vi "Host.vi"() -> ()   [LabVIEW 2018]
uses:
  <instrlib>/niDCPower/nidcpower.llb/niDCPower Measurement Type.ctl
  <vilib>/FPGAPlugInAG/PXI-7953R/niLvFpga_Open_PXI-7953R.vi
  <vilib>/rvi/interface/common/dynamic/niFpgaDynamicAddResources.vi
  <vilib>/FPGAPlugInAG/Dynamic/niLvFpga_Reset_Dynamic.vi
  <vilib>/FPGAPlugInAG/Dynamic/niLvFpga_Run_Dynamic.vi
  <vilib>/Utility/error.llb/Error Cluster From Error Code.vi
  <vilib>/rvi/errors/niLvFpgaAdjustHostInterfaceError.vi
  <vilib>/FPGAPlugInAG/Dynamic/niLvFpga_Close_Dynamic.vi
  <vilib>/rvi/interface/nirviOpenFPGA/nirviOpenFPGA.xnode
  FPGA Bitfiles/EV76C661aab_FPGATarget_Target_Ci7Vxfb6PyU.lvbitx
  <vilib>/rvi/interface/nirviMethod/nirviMethod.xnode
  <vilib>/rvi/interface/nirviReadWriteControl/nirviReadWriteControl.xnode
  <vilib>/rvi/interface/nirviCloseFPGA/nirviCloseFPGA.xnode
  NiFpgaLv.dll
  <vilib>/rvi/interface/Simulation/niFpgaSimulationCallBeginRW.vi
  <vilib>/FPGAPlugInAG/Dynamic/niLvFpga_ReadFifo_Dynamic.vi
  <vilib>/rvi/errors/niLvFpgaMergeErrorWithErrorCode.vi
panel:
  in  "Tab Control":enum32{"Панель управления", "Панель отладки"}(tab)
  in  "Frames":path=path "D:/NI LabVIEW/EV76C661_aab/Frames"
  out "CountFIFO":u32
  out "AddCounter":u32
  in  "Сохранить":bool
  in  "Темный(F)\nСветлый(T)":bool
  in  "Примечание":string
  out "Image":T1(plugin-control)
  in  "Непрерывно":bool
  in  "Получить кадр":bool
  out "Last SEU Time":string
  out "Reg Counter":u8
  in  "SEU":path=path "D:/NI LabVIEW/EV76C661_aab/SEU"
  out "Счетчик сбоев":u16
  in  "Содержание всех регистров":u16[](array[numeric])=[1, 0, 0, 0, 32880, 0, 53338, 2561, 56097, 24869, 512, 260, 0, 0, 512, 0, 0, 0, 6, 1024, 6, 1280, 0, 0, 0, 0, 0, 512, 0, 0, 0, 6, 1024, 6, 1280, 0, 512, 0, 0, 0, 6, 1024, 6, 1280, 0, 512, 0, 0, 0, 6, 1024, 6, 1280, 0, 32896, 32896, 0, 14464, 32960, 0, 0, 0, 0, 0, 0, 0, 0, 0, 8192, 0, 0, 0, 0, 31601, 0, 0, 0, 0, 0, 0, 0, 0, 0, 0, 0, 0, 0, 0, 0, 0, 0, 0, 0, 0, 0, 0, 0, 0, 0, 0, 0, 0, 0, 0, 0, 0, 0, 0, 0, 0, 0, 0, 0, 0, 0, 0, 0, 0, 0, 0, 0, 0, 0, 0, 0, 0, 0, 2048]
  in  "Регистры для записи":u16[](array[numeric])=[2561, 56217, 24976, 512, 260, 512]
  in  "Проверка\nсбоев":bool
  in  "Прошить\nрегистры":bool
  in  "TRIG":bool
  in  "Автомат":bool
  in  "SIM_SEL":bool
  in  "VDD18D_selcur, A":dbl=0.06 caption="current limit" format="%_6p"
  in  "VDD18A_selcur, A":dbl=0.05 caption="current limit" format="%_6p"
  in  "VDD33A_selcur, A":dbl=0.06 caption="current limit" format="%_6p"
  out "VDD18A_counter":u32
  out "VDD33A_counter":u32
  out "VDD18D_counter":u32
  out "VDD18A_SEL_warning":bool
  out "VDD33A_SEL_warning":bool
  out "VDD18D_SEL_warning":bool
  in  "STOP":bool
  in  "Power":bool
  in  "VDD18D, V":dbl=1.8 caption="voltage level" format="%_6p"
  in  "VDD18D_curlim, A":dbl=0.1 caption="current limit" format="%_6p"
  in  "VDD18A_curlim, A":dbl=0.1 caption="current limit" format="%_6p"
  out "VDD18D_cur, A":dbl caption="measurement" format="%_6g"
  out "VDD18A_cur, A":dbl caption="measurement" format="%_6g"
  in  "VDD18A, V":dbl=1.7999999999999985 caption="voltage level" format="%_6p"
  out "VDD18D_char":dbl(graph)=-0.006831291044701817
  out "VD18A_char":dbl(graph)=-2.772283562549262e-06
  in  "VDD33A_curlim, A":dbl=0.1 caption="current limit" format="%_6p"
  out "VDD33A_cur, A":dbl caption="measurement" format="%_6g"
  in  "VDD33A, V":dbl=3.300000000000001 caption="voltage level" format="%_6p"
  out "VDD18A_char":dbl(graph)=4.6397717644130316e-05
  in  "VDD33A_VDD18A":refnum<k15>="PXI1Slot2_2"
  in  "VDD18D":refnum<k15>="PXI1Slot3_3"
  in  "FPGA":tag="RIO0"
  in  "SEL":path=path "D:/NI LabVIEW/EV76C661_aab/SEL"
  out "№":string
  out "Default":string
  out "During SEU":string
  in  "Кадр готов":bool
  out "MISO":bool[](array[boolean])
  out "DataTime":u32
  out "DelayFrame":u32
  in  "WatchDogTime":u32=5000
  out "DataFailure":bool
  out "MOSI":bool[](array[boolean])
  out "Образец №":string="1"
  in  "NumberOfAdd":u32=1310720
  out "DataToFrame":u16[][](array[numeric])
  out "SEL":bool
  out "Сбой":bool
  in  "CSN в конце по С(F)/Ф(T)":bool
  in  "Чтение по С(F)/Ф(T)":bool=TRUE
  in  "Маска номера":i32[](array[numeric])=[0, -1, 2, 3, 4, 5, 6, 7, 8, 9, 10, 11, 12, 13, 14, 15, 16, 17, 18, 19, 20, 21, 22, 23, 24, 25, 26, 27, 28, 29, 30, 31, 32, 33, 34, 35, 36, 37, 38, 39, 40, 41, 42, 43, 44, 45, 46, 47, 48, 49, 50, 51, 52, 53, 54, 55, 56, 57, 58, 59, -1, -1, -1, -1, -1, -1, -1, -1, -1, -1, -1, -1, -1, -1, -1, -1, -1, -1, -1, -1, -1, -1, -1, -1, -1, -1, -1, -1, -1, -1, -1, -1, -1, -1, -1, -1, -1, -1, -1, -1, -1, -1, -1, -1, -1, -1, -1, -1, -1, -1, -1, -1, -1, -1, -1, -1, -1, -1, -1, -1, -1, -1, -1, -1, -1, -1, -1, 127, 0, 0, 0, 0, 0, 0, 0, 0, 0, 0, 0, 0, 0, 0, 0, 0, 0, 0, 0, 0, 0, 0, 0, 0, 0, 0, 0, 0, 0, 0, 0, 0, 0, 0, 0, 0, 0, 0, 0, 0, 0, 0, 0, 0, 0, 0, 0, 0, 0, 0, 0, 0, 0, 0, 0, 0, 0, 0, 0, 0, 0, 0, 0, 0, 0, 0, 0, 0, 0, 0, 0, 0, 0, 0, 0, 0, 0, 0, 0, 0, 0, 0, 0, 0, 0, 0, 0, 0, 0, 0, 0, 0, 0, 0, 0, 0, 0, 0, 0, 0, 0, 0, 0, 0, 0, 0, 0, 0, 0, 0, 0, 0, 0, 0, 0, 0, 0, 0, 0, 0, 0, 0, 0, 0, 0, 0, 0, 0]
  in  "Номера для Записи":u32[](array[numeric])=[7, 8, 9, 10, 11, 14]
  in  "Такт чтения после адреса":u8=1
  in  "27_STOP":u8=27
  in  "19_STOP":u8=19
  out "Power OFF":bool
  in  "Делитель 24/x":u8=2
  in  "RESET":bool
  in  "Wait_parry, ms":u32=100
  in  "VDD33_ON":bool
  in  "VDD18_ON":bool
  in  "TrigTime":u32=500
  in  "Retrieve":u8
  in  "Request":u8
  out "SPI":bool
  in  "SPI_Write":bool
  out "WriteIsDone":bool
  in  "SPI_Read":bool
  out "DataRead":u16
  in  "RegForRead":u8
  in  "RegForWrite":u8
  in  "DataWrite":u16
  out "ReadIsDone":bool
  out "FirmwareIsDone":bool
  # "0 - 7       h07\n1 - 8       h08\n2 - 9       h09\n3 - 10     h0A\n4 - 11     h0B\n5 - 14     h0E"
  # "h08\n56217\n56319"
  # "h09\n24960\n24976"
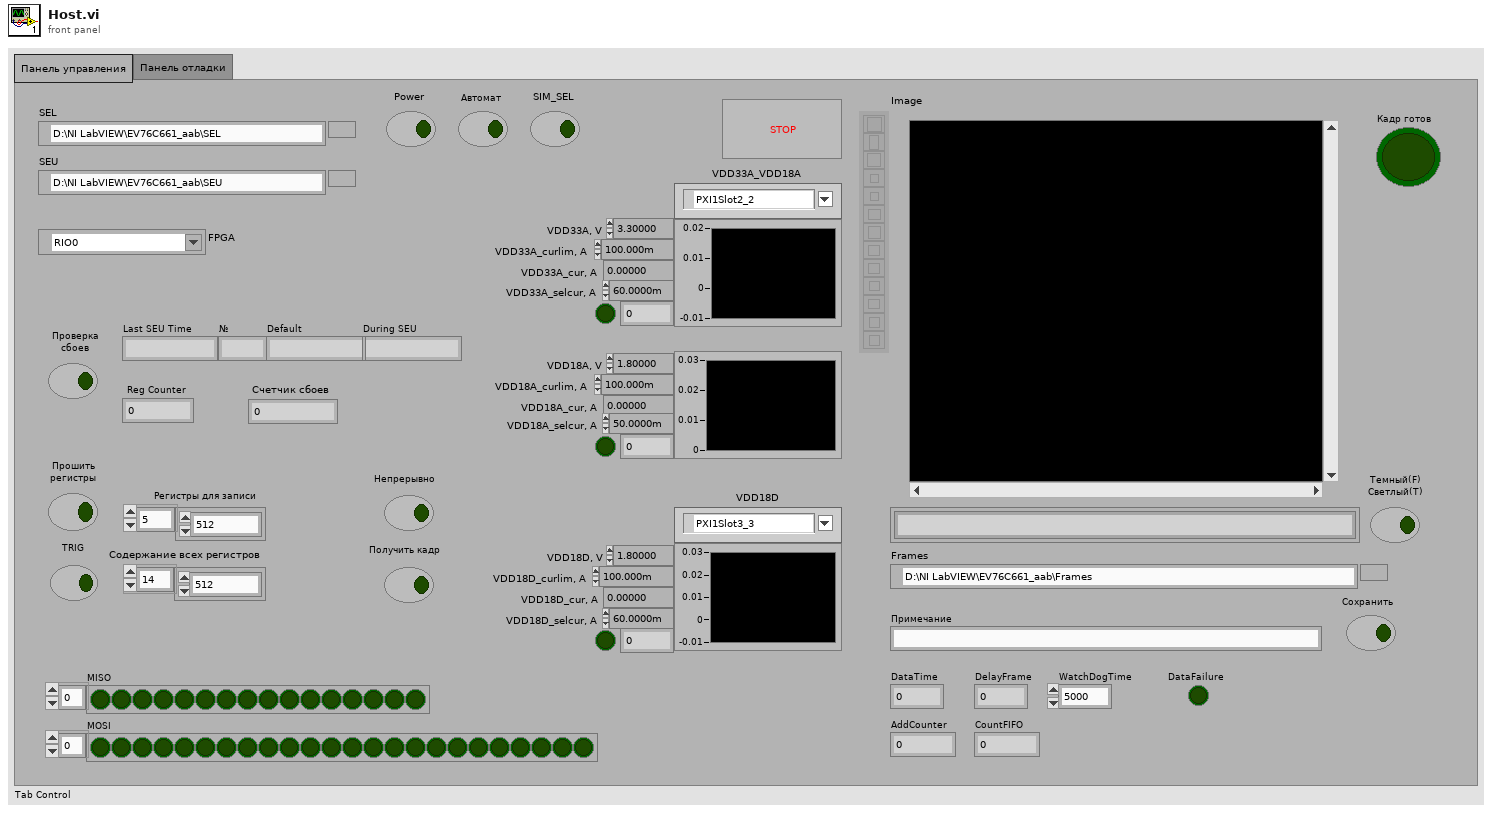
[diagram p1: front panel]
types:
  T1 = typedef "IMAQ Image.ctl" = refnum<image>
  T2 = enum16{"open", "replace", "create", "open or create", "replace or create", "replace or create with confirmation"}
  T3 = typedef "Image Type" = u32
  T4 = typedef "niDCPower Measurement Type.ctl" = i32
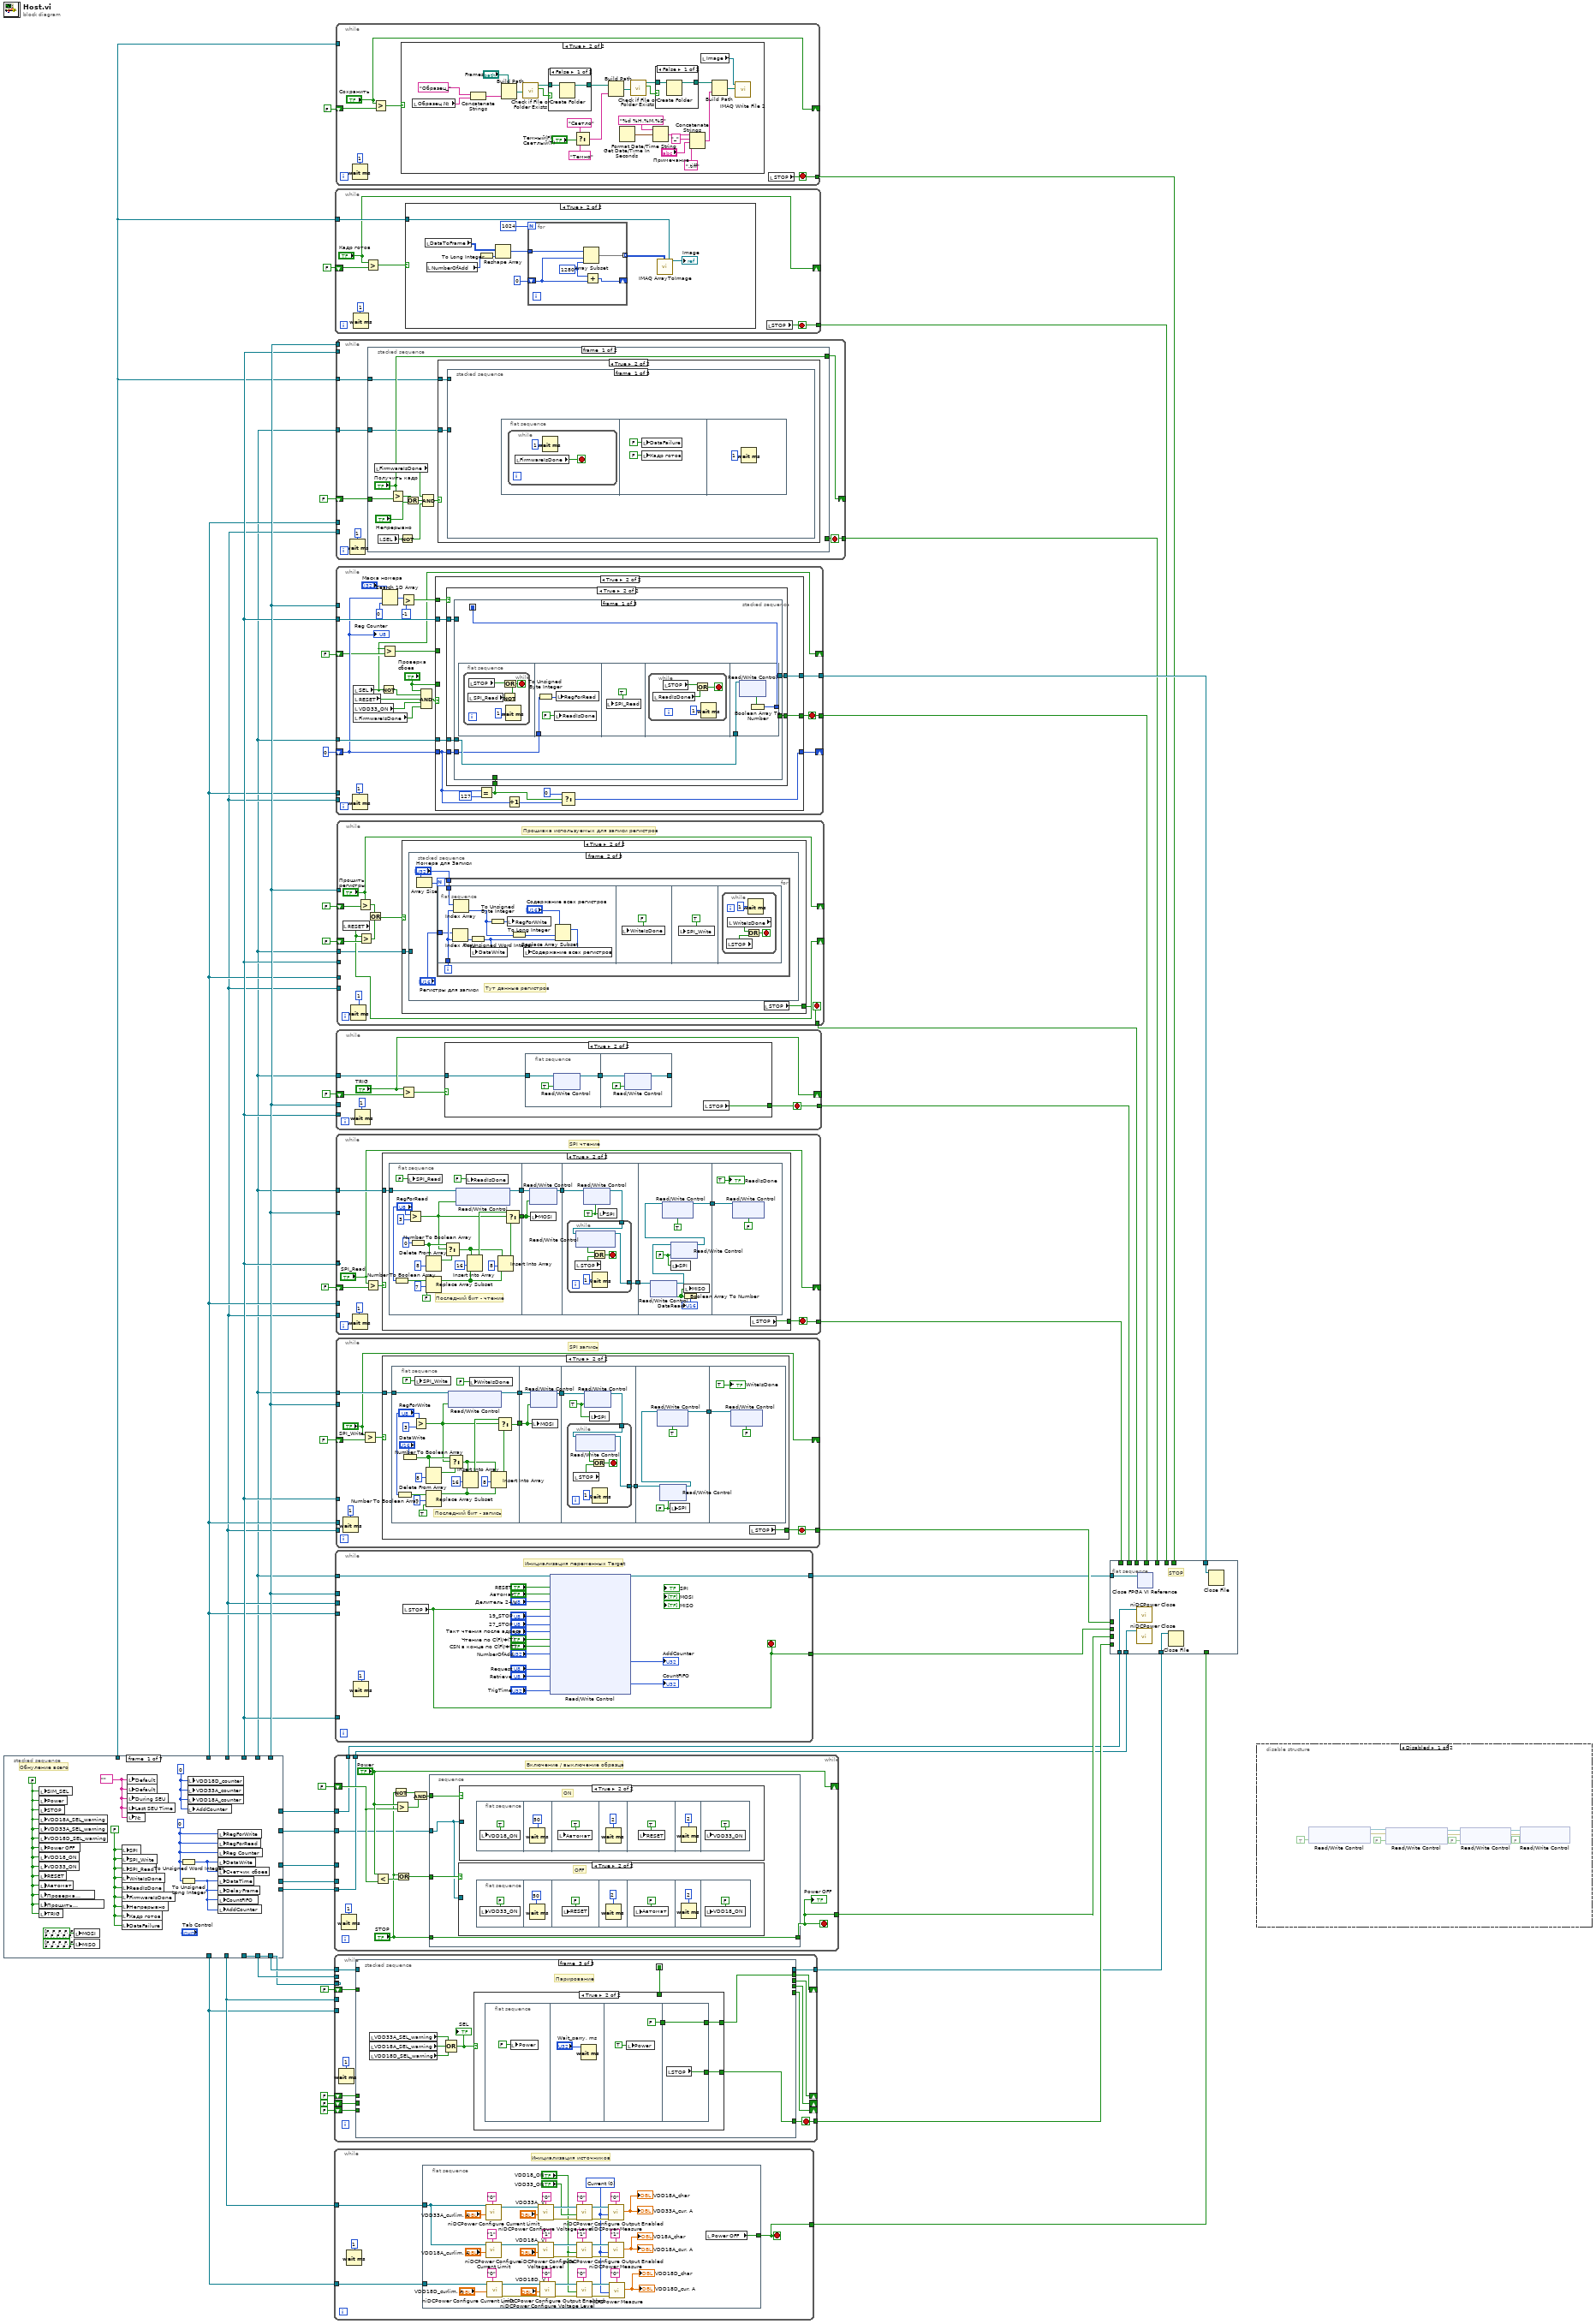
[diagram p0: block diagram]
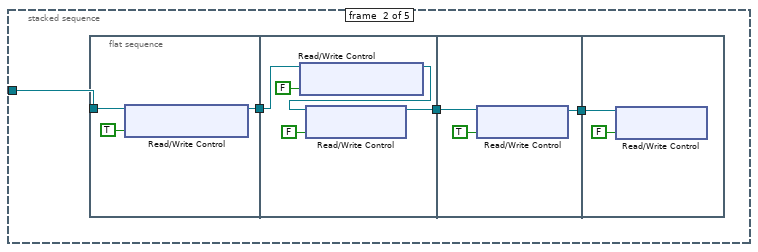
[diagram p8: hidden frame]
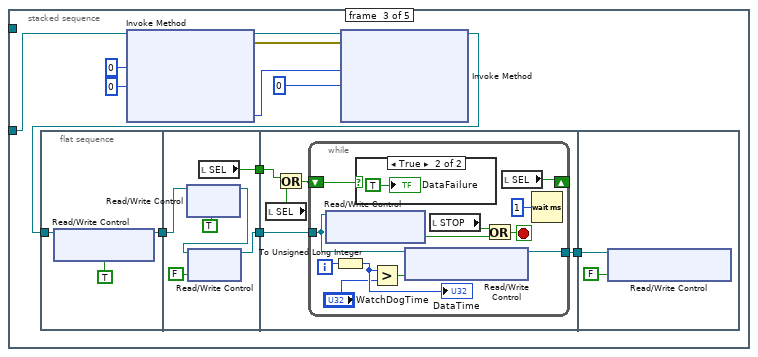
[diagram p9: hidden frame]
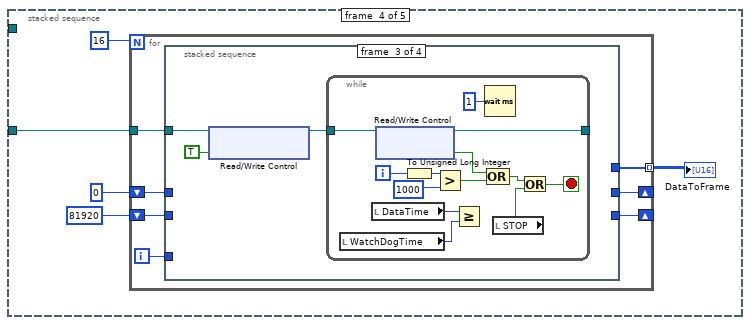
[diagram p11: hidden frame]
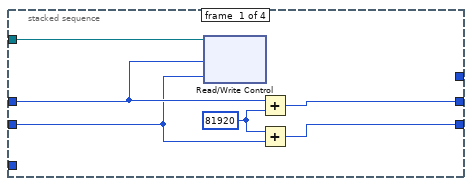
[diagram p12: hidden frame]
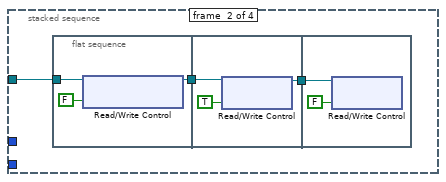
[diagram p13: hidden frame]
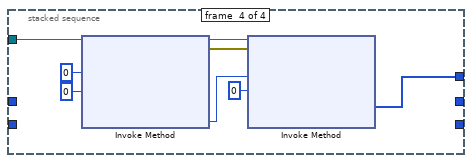
[diagram p14: hidden frame]
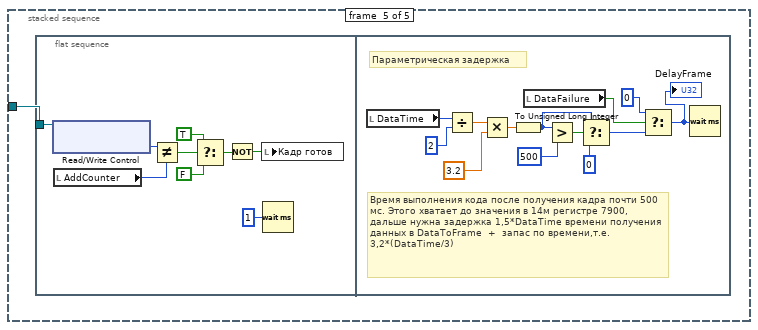
[diagram p15: hidden frame]
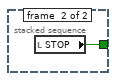
[diagram p16: hidden frame]
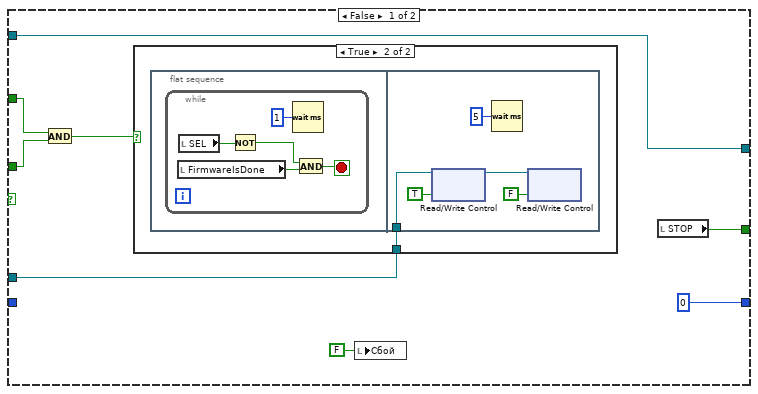
[diagram p17: hidden frame]
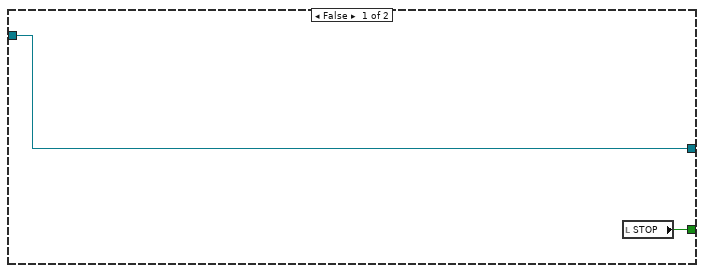
[diagram p19: hidden frame]
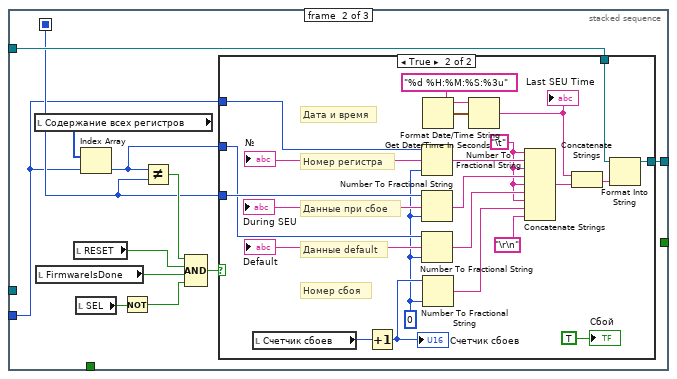
[diagram p20: hidden frame]
diagram:
  n1 = stacked-sequence {
    tunnel: [_ _ _ _ _ w121 _] -> w45
    tunnel: [_ _ _ _ _ w120 _] -> w46
    tunnel: [_ _ w62 _ _ _ _] -> w47
    tunnel: [_ _ _ _ w114 _ _] -> w36
    tunnel: [_ _ _ _ w114 _ _] -> w2
    tunnel: [_ _ _ _ w114 _ _] -> w38
    tunnel: [_ _ _ _ _ w120 _] -> w30
    tunnel: [_ _ _ _ _ w121 _] -> w31
    tunnel: [_ _ _ _ _ w121 _] -> w12
    tunnel: [_ _ _ _ _ w120 _] -> w13
    tunnel: [_ _ w62 _ _ _ _] -> w15
    tunnel: [_ _ w62 _ _ _ _] -> w37
    tunnel: [_ _ _ w87 _ _ _] -> w18
    tunnel: [_ _ _ w87 _ _ _] -> w14
    tunnel: [_ _ _ w87 _ _ _] -> w17
    tunnel: [_ _ _ _ _ _ w132] -> w3
    frame #0 {
      w49 = "" ("Last SEU Data")
      w55 = u32 0 ("VDD18D_counter")
      w54 = u8 0
      w53 = FALSE
      w57 = FALSE
      # "Обнуление всего"
      n2 = local write "SIM_SEL"(w57) -> ()
      n3 = local write "Power"(w57) -> ()
      n4 = local write "STOP"(w57) -> ()
      n5 = local write "VDD18A_SEL_warning"(w57) -> ()
      n6 = local write "VDD33A_SEL_warning"(w57) -> ()
      n7 = local write "VDD18D_SEL_warning"(w57) -> ()
      n8 = local write "Power OFF"(w57) -> ()
      n9 = local write "VDD18_ON"(w57) -> ()
      n10 = local write "VDD33_ON"(w57) -> ()
      n11 = local write "RESET"(w57) -> ()
      n12 = local write "Автомат"(w57) -> ()
      n13 = local write "Проверка\nсбоев"(w57) -> ()
      n14 = local write "Прошить\nрегистры"(w57) -> ()
      n15 = local write "TRIG"(w57) -> ()
      n16 = local write "MOSI"(bool[] [FALSE, FALSE, FALSE, FALSE, FALSE, FALSE, FALSE, FALSE, FALSE, FALSE, FALSE, FALSE, FALSE, FALSE, FALSE, FALSE, FALSE, FALSE, FALSE, FALSE, FALSE, FALSE, FALSE, FALSE] ("MOSI")) -> ()
      n17 = local write "MISO"(bool[] [FALSE, FALSE, FALSE, FALSE, FALSE, FALSE, FALSE, FALSE, FALSE, FALSE, FALSE, FALSE, FALSE, FALSE, FALSE, FALSE] ("MISO")) -> ()
      n18 = local write "SPI"(w53) -> ()
      n19 = local write "SPI_Write"(w53) -> ()
      n20 = local write "SPI_Read"(w53) -> ()
      n21 = local write "WriteIsDone"(w53) -> ()
      n22 = local write "ReadIsDone"(w53) -> ()
      n23 = local write "FirmwareIsDone"(w53) -> ()
      n24 = local write "Непрерывно"(w53) -> ()
      n25 = local write "Кадр готов"(w53) -> ()
      n26 = local write "DataFailure"(w53) -> ()
      n27 = local write "Default"(w49) -> ()
      n28 = local write "Default"(w49) -> ()
      n29 = local write "During SEU"(w49) -> ()
      n30 = local write "Last SEU Time"(w49) -> ()
      n31 = local write "№"(w49) -> ()
      n32 = To Unsigned Word Integer(number=w54) -> (unsigned 16bit integer=w56:u16)
      n33 = To Unsigned Long Integer(number=w54) -> (unsigned 32bit integer=w52:u32)
      n34 = local write "VDD18D_counter"(w55) -> ()
      n35 = local write "VDD33A_counter"(w55) -> ()
      n36 = local write "VDD18A_counter"(w55) -> ()
      n37 = local write "AddCounter"(w55) -> ()
      n38 = local write "RegForWrite"(w54) -> ()
      n39 = local write "RegForRead"(w54) -> ()
      n40 = local write "Reg Counter"(w54) -> ()
      n41 = local write "DataWrite"(w56) -> ()
      n42 = local write "Счетчик сбоев"(w56) -> ()
      n43 = local write "DataTime"(w52) -> ()
      n44 = local write "DelayFrame"(w52) -> ()
      n45 = local write "CountFIFO"(w52) -> ()
      n46 = local write "AddCounter"(w52) -> ()
    }
    frame #1 {
      n47 = call "Begin.vi"() -> ("Образец № 2"=→"Образец №":string)  [unwired: 9 in]
    }
    frame #2 {
      w60 = "\t"
      # "Инициализация файла"
      n48 = local read "Образец №"() -> (w61:string)
      n49 = Build Path(base path="SEL", name or relative path=w61) -> (appended path=w82:path)
      n50 = Get Date/Time In Seconds() -> (seconds since 1Jan1904=w78:timestamp)
      n51 = call <vilib>:"Check if File or Folder Exists.vi"("path"=w82) -> ("file or folder exists?"=w81:bool, "dup path"=w80:path)  [unwired: 8 in, 1 out]
      n52 = Format Date/Time String(time format string (%c)="%d %H.%M.%S", seconds (now)=w78) -> (date/time string=w77:string)  [unwired: 1 in]
      n53 = case shown="False" w81 {
        tunnel: w80 -> [w84 w85]
        tunnel: [w83 w85] -> w79
        frame False {
          n54 = Create Folder(path (use dialog)=w84) -> (created path=w83:path)  [unwired: 2 in, 2 out]
        }
        frame True {
        }
      }
      n55 = Concatenate Strings(w77, ".xls" ("string")) -> (w74:string)
      n56 = Build Path(base path=w79, name or relative path=w74) -> (appended path=w71:path)
      n57 = Open/Create/Replace File(file path (use dialog)=w71, operation (0:open)=T2."open or create", access (0:read/write)=enum16{"read/write", "read-only", "write-only"}."read/write") -> (refnum out=w66:refnum<file>)  [unwired: 3 in, 2 out]
      n58 = Set File Position(refnum=w66, from (0:start)=enum16{"start", "end", "current"}."end") -> (refnum out=w64:refnum<file>)  [unwired: 2 in, 1 out]
      n59 = Format Into String(initial string=w64, "Time" ("string"), w60, "VD33A" ("string"), w60, "VD18A" ("string"), w60, "VD18D" ("string"), w60, "\r\n") -> (resulting string=w62:refnum<file>)  [unwired: 2 in, 1 out]
    }
    frame #3 {
      w90 = "\t"
      # "Инициализация файла"
      n60 = local read "Образец №"() -> (w86:string)
      n61 = Build Path(base path="SEU", name or relative path=w86) -> (appended path=w110:path)
      n62 = Get Date/Time In Seconds() -> (seconds since 1Jan1904=w106:timestamp)
      n63 = call <vilib>:"Check if File or Folder Exists.vi"("path"=w110) -> ("file or folder exists?"=w109:bool, "dup path"=w108:path)  [unwired: 8 in, 1 out]
      n64 = Format Date/Time String(time format string (%c)="%d %H.%M.%S", seconds (now)=w106) -> (date/time string=w105:string)  [unwired: 1 in]
      n65 = case shown="False" w109 {
        tunnel: w108 -> [w112 w113]
        tunnel: [w111 w113] -> w107
        frame False {
          n66 = Create Folder(path (use dialog)=w112) -> (created path=w111:path)  [unwired: 2 in, 2 out]
        }
        frame True {
        }
      }
      n67 = Concatenate Strings(w105, ".xls" ("string")) -> (w104:string)
      n68 = Build Path(base path=w107, name or relative path=w104) -> (appended path=w103:path)
      n69 = Open/Create/Replace File(file path (use dialog)=w103, operation (0:open)=T2."open or create", access (0:read/write)=enum16{"read/write", "read-only", "write-only"}."read/write") -> (refnum out=w102:refnum<file>)  [unwired: 3 in, 2 out]
      n70 = Set File Position(refnum=w102, from (0:start)=enum16{"start", "end", "current"}."end") -> (refnum out=w101:refnum<file>)  [unwired: 2 in, 1 out]
      n71 = Format Into String(initial string=w101, "Time" ("string"), w90, "Reg№" ("string"), w90, "Data now" ("string"), w90, "Data default" ("input 7"), w90, "Counter" ("input 9"), "\r\n") -> (resulting string=w87:refnum<file>)  [unwired: 2 in, 1 out]
    }
    frame #4 {
      # "Подключение FPGA"
      n72 = xnode "Open FPGA VI Reference"("resource name"="FPGA") -> ("FPGA VI Reference Out"=w118:refnum<k20>, "error out"=w116:errorcluster)  [unwired: 1 in]
      n73 = xnode "Invoke Method"("FPGA VI Reference In"=w118, "error in"=w116) -> ("FPGA VI Reference Out"=w115:refnum<k20>, "error out"=w117:errorcluster)
      n74 = xnode "Invoke Method"("FPGA VI Reference In"=w115, "error in"=w117) -> ("FPGA VI Reference Out"=w114:refnum<k20>)  [unwired: 1 in, 1 out]
    }
    frame #5 {
      # "Инициализация источников"
      n75 = call <instrlib>:"niDCPower Initialize.vi"("resource name"="VDD33A_VDD18A") -> ("error out"=w126:errorcluster, "instrument handle out"=w128:refnum<k15>)  [unwired: 3 in, 6 out]
      n76 = call <instrlib>:"niDCPower Initialize.vi"("resource name"="VDD18D") -> ("error out"=w127:errorcluster, "instrument handle out"=w129:refnum<k15>)  [unwired: 3 in, 6 out]
      n77 = call <instrlib>:"niDCPower Configure Voltage Level.vi"("error in (no error)"=w126, "voltage level"=0.0, "channel name"="0,1", "instrument handle"=w128) -> ("instrument handle out"=w121:refnum<k15>)  [unwired: 6 in, 1 out]
      n78 = call <instrlib>:"niDCPower Configure Voltage Level.vi"("error in (no error)"=w127, "voltage level"=0.0, "channel name"="0", "instrument handle"=w129) -> ("instrument handle out"=w120:refnum<k15>)  [unwired: 6 in, 1 out]
    }
    frame #6 {
      w133 = T3 7 items=["Grayscale (U8)", "Grayscale (I16)", "Grayscale (SGL)", "Complex (CSG)", "RGB (U32)", "HSL (U32)", "RGB (U64)", "Grayscale (U16)"] ("Image Type")
      n79 = call "IMAQ Create"("Image Name"="EV76C661", "Image Type"=w133) -> ("New Image"=w132:T1)  [unwired: 3 in, 1 out]
    }
  }
  n80 = while {
    tunnel: w45 -> [w137]
    tunnel: w46 -> [w136]
    shift-right: ["Power"] -> _
    shift-left: FALSE ("Питание") -> [w146]
    tunnel: w38 -> [w135]
    tunnel: w37 -> [_]
    tunnel: [w138] -> w29
    tunnel: w17 -> [_]
    tunnel: [w137] -> w8
    tunnel: [w136] -> w7
    stop <- w138 stop-if-true
    # "Включение / выключение образца"
    n81 = Wait (ms)(milliseconds to wait=u32 1) -> ()  [unwired: 1 out]
    n82 = Less?(x="Power", y=w146) -> (x < y?=w141:bool)
    n83 = Not(x="STOP") -> (.not. x?=w143:bool)
    n84 = Greater?(x="Power", y=w146) -> (0:w142:bool)
    n85 = Or(x="STOP", y=w141) -> (x .or. y?=w140:bool)
    n86 = And(x=w143, y=w142) -> (x .and. y?=w144:bool)
    n87 = stacked-sequence {
      tunnel: w144 -> [w151]
      tunnel: w140 -> [w150]
      tunnel: [w149] -> w138
      tunnel: "STOP" -> [w149]
      tunnel: w135 -> [w148]
      frame #0 {
        n88 = case shown="True" w150 {
          tunnel: w148 -> [_ _]
          frame False {
          }
          frame True {
            # "OFF"
            n89 = flat-sequence {
              frame #0 {
                n90 = local write "VDD33_ON"(FALSE ("VDD18_ON")) -> ()
              }
              frame #1 {
                n91 = Wait (ms)(milliseconds to wait=u32 50) -> ()  [unwired: 1 out]
              }
              frame #2 {
                n92 = local write "RESET"(FALSE ("VDD18_ON")) -> ()
              }
              frame #3 {
                n93 = Wait (ms)(milliseconds to wait=u32 2) -> ()  [unwired: 1 out]
              }
              frame #4 {
                n94 = local write "Автомат"(FALSE ("VDD18_ON")) -> ()
              }
              frame #5 {
                n95 = Wait (ms)(milliseconds to wait=u32 2) -> ()  [unwired: 1 out]
              }
              frame #6 {
                n96 = local write "VDD18_ON"(FALSE ("VDD18_ON")) -> ()
              }
            }
          }
        }
        n97 = case shown="True" w151 {
          tunnel: w148 -> [_ _]
          frame False {
          }
          frame True {
            # "ON"
            n98 = flat-sequence {
              frame #0 {
                n99 = local write "VDD18_ON"(TRUE ("VDD18_ON")) -> ()
              }
              frame #1 {
                n100 = Wait (ms)(milliseconds to wait=u32 50) -> ()  [unwired: 1 out]
              }
              frame #2 {
                n101 = local write "Автомат"(TRUE ("VDD18_ON")) -> ()
              }
              frame #3 {
                n102 = Wait (ms)(milliseconds to wait=u32 2) -> ()  [unwired: 1 out]
              }
              frame #4 {
                n103 = local write "RESET"(TRUE ("VDD18_ON")) -> ()
              }
              frame #5 {
                n104 = Wait (ms)(milliseconds to wait=u32 2) -> ()  [unwired: 1 out]
              }
              frame #6 {
                n105 = local write "VDD33_ON"(TRUE ("VDD18_ON")) -> ()
              }
            }
          }
        }
      }
    }
    "Power OFF" <- w138
  }
  n106 = while {
    shift-right: [w167] -> _
    shift-left: FALSE ("Питание") -> [w178]
    tunnel: w47 -> [w176]
    tunnel: w30 -> [_]
    tunnel: w31 -> [_]
    tunnel: [w175] -> w44
    tunnel: [w174] -> w43
    shift-right: [w168] -> _
    shift-left: FALSE ("Питание") -> [w173]
    shift-right: [w169] -> _
    shift-left: FALSE ("Питание") -> [w172]
    shift-right: [w170] -> _
    shift-left: FALSE ("Питание") -> [w171]
    tunnel: w36 -> [_]
    tunnel: [w166] -> _
    tunnel: w18 -> [w166]
    stop <- w175 stop-if-true
    n107 = Wait (ms)(milliseconds to wait=u32 1) -> ()  [unwired: 1 out]
    n108 = stacked-sequence {
      seq-local: [w179 _ _] -> [_ _ w264]
      tunnel: w178 -> [w193 _ _]
      tunnel: [_ _ w269] -> w175
      tunnel: w176 -> [_ w246 _]
      tunnel: [_ w245 _] -> w174
      tunnel: w173 -> [w190 _ _]
      tunnel: w172 -> [w187 _ _]
      tunnel: w171 -> [w185 _ _]
      tunnel: [w182 _ _] -> w170
      tunnel: [w181 _ _] -> w169
      tunnel: [w180 _ _] -> w168
      tunnel: [_ _ w265] -> w167
      frame #0 {
        # "Детектирование SEL"
        n109 = local read "Power"() -> (w179:bool)
        n110 = Greater?(x=w179, y=w193) -> (0:w192:bool)
        n111 = flat-sequence {
          tunnel: w192 -> [w194]
          tunnel: [w197] -> w191
          tunnel: w190 -> [w197]
          tunnel: [w196] -> w188
          tunnel: w187 -> [w196]
          tunnel: w185 -> [w195]
          tunnel: [w195] -> w183
          tunnel: [w205] -> w180
          tunnel: [w204] -> w181
          tunnel: [w203] -> w182
          tunnel: w191 -> [w202]
          tunnel: [w202] -> w189
          tunnel: w188 -> [w201]
          tunnel: [w201] -> w186
          tunnel: [w200] -> w184
          tunnel: w183 -> [w200]
          tunnel: w189 -> [w217]
          tunnel: w186 -> [w216]
          tunnel: w184 -> [w215]
          frame #0 {
            # "Защита от первичного качка напряжения\n(чтобы счетчик не посчитал лишнее событие)"
            n112 = case shown="False" w194 {
              frame False {
              }
              frame True {
                n113 = Wait (ms)(milliseconds to wait=u32 500) -> ()  [unwired: 1 out]
              }
            }
          }
          frame #1 {
            n114 = local read "VDD18D_cur, A"() -> (w214:dbl)
            n115 = local read "VDD18A_cur, A"() -> (w213:dbl)
            n116 = local read "VDD33A_cur, A"() -> (w212:dbl)
            n117 = Greater Or Equal?(x=w214, y="VDD18D_selcur, A") -> (x >= y?=w206:bool)
            n118 = Greater Or Equal?(x=w213, y="VDD18A_selcur, A") -> (x >= y?=w208:bool)
            n119 = Greater Or Equal?(x=w212, y="VDD33A_selcur, A") -> (x >= y?=w207:bool)
            n120 = Or(x="SIM_SEL", y=w206) -> (x .or. y?=w205:bool)
            "VDD18A_SEL_warning" <- w205
            n121 = Or(x="SIM_SEL", y=w207) -> (x .or. y?=w203:bool)
            "VDD18D_SEL_warning" <- w203
            n122 = Or(x="SIM_SEL", y=w208) -> (x .or. y?=w204:bool)
            "VDD33A_SEL_warning" <- w204
          }
          frame #2 {
            n123 = local read "VDD18A_SEL_warning"() -> (w218:bool)
            n124 = local read "VDD33A_SEL_warning"() -> (w219:bool)
            n125 = local read "VDD18D_SEL_warning"() -> (w220:bool)
            n126 = local read "SIM_SEL"() -> (w221:bool)
            n127 = Greater?(x=w218, y=w217) -> (0:w223:bool)
            n128 = Greater?(x=w219, y=w216) -> (0:w224:bool)
            n129 = Greater?(x=w220, y=w215) -> (0:w225:bool)
            n130 = Not(x=w221) -> (.not. x?=w222:bool)
            n131 = And(x=w223, y=w222) -> (x .and. y?=w228:bool)
            n132 = And(x=w224, y=w222) -> (x .and. y?=w227:bool)
            n133 = And(x=w225, y=w222) -> (x .and. y?=w226:bool)
            n134 = case shown="True" w228 {
              frame False {
              }
              frame True {
                n135 = local read "VDD18A_counter"() -> (w232:u32)
                n136 = Increment(x=w232) -> (x+1=→"VDD18A_counter":u32)
              }
            }
            n137 = case shown="True" w227 {
              frame False {
              }
              frame True {
                n138 = local read "VDD33A_counter"() -> (w230:u32)
                n139 = Increment(x=w230) -> (x+1=→"VDD33A_counter":u32)
              }
            }
            n140 = case shown="True" w226 {
              frame False {
              }
              frame True {
                n141 = local read "VDD18D_counter"() -> (w233:u32)
                n142 = Increment(x=w233) -> (x+1=→"VDD18D_counter":u32)
              }
            }
          }
        }
      }
      frame #1 {
        w258 = 0
        w259 = 6
        w240 = "\t"
        # "Запись логов"
        n143 = local read "VDD33A_SEL_warning"() -> (w244:bool)
        n144 = local read "VDD18A_SEL_warning"() -> (w243:bool)
        n145 = local read "VDD18D_SEL_warning"() -> (w242:bool)
        n146 = local read "VDD33A_cur, A"() -> (w255:dbl)
        n147 = local read "VDD18A_cur, A"() -> (w254:dbl)
        n148 = local read "VDD18D_cur, A"() -> (w253:dbl)
        n149 = local read "VDD33A_counter"() -> (w252:u32)
        n150 = local read "VDD18A_counter"() -> (w251:u32)
        n151 = local read "VDD18D_counter"() -> (w250:u32)
        n152 = Get Date/Time In Seconds() -> (seconds since 1Jan1904=w262:timestamp)
        n153 = Format Date/Time String(time format string (%c)="%d %H:%M:%S:%3u", seconds (now)=w262) -> (date/time string=w260:string)  [unwired: 1 in]
        n154 = Number To Fractional String(number=w255, width (-)=w259, precision (6)=w259) -> (F-format string=w249:string)  [unwired: 1 in]
        n155 = Number To Fractional String(number=w254, width (-)=w259, precision (6)=w259) -> (F-format string=w248:string)  [unwired: 1 in]
        n156 = Number To Fractional String(number=w253, width (-)=w259, precision (6)=w259) -> (F-format string=w241:string)  [unwired: 1 in]
        n157 = Number To Fractional String(number=w252, width (-)=w258, precision (6)=w258) -> (F-format string=w239:string)  [unwired: 1 in]
        n158 = Number To Fractional String(number=w251, width (-)=w258, precision (6)=w258) -> (F-format string=w238:string)  [unwired: 1 in]
        n159 = Number To Fractional String(number=w250, width (-)=w258, precision (6)=w258) -> (F-format string=w237:string)  [unwired: 1 in]
        n160 = Compound Arithmetic op=OR(w244, w243, w242) -> (w257:bool)
        n161 = Select(t="!!!", s=w257, f="") -> (s? t:f=w236:string)
        n162 = Concatenate Strings(w260, w240, w249, w240, w248, w240, w241, w240, w239, w240, w238, w240, w237, w240, w236, "\r\n") -> (w247:string)
        n163 = Format Into String(initial string=w246, w247) -> (resulting string=w245:refnum<file>)  [unwired: 2 in, 1 out]
      }
      frame #2 {
        # "Парирование"
        n164 = local read "VDD33A_SEL_warning"() -> (w266:bool)
        n165 = local read "VDD18A_SEL_warning"() -> (w268:bool)
        n166 = local read "VDD18D_SEL_warning"() -> (w267:bool)
        n167 = Compound Arithmetic op=OR(w266, w268, w267) -> (w270:bool)
        "SEL" <- w270
        n168 = case shown="True" w270 {
          tunnel: [w272 w275] -> w269
          tunnel: [w271 w274] -> w265
          tunnel: w264 -> [w271 _]
          frame False {
            n169 = local read "STOP"() -> (w272:bool)
          }
          frame True {
            n170 = flat-sequence {
              tunnel: [FALSE] -> w273
              tunnel: [w281] -> w275
              tunnel: [w280] -> w274
              tunnel: w273 -> [w280]
              frame #0 {
                n171 = local write "Power"(FALSE ("Power")) -> ()
              }
              frame #1 {
                n172 = Wait (ms)(milliseconds to wait="Wait_parry, ms") -> ()  [unwired: 1 out]
              }
              frame #2 {
                n173 = local write "Power"(TRUE ("Power")) -> ()
              }
              frame #3 {
                n174 = local read "STOP"() -> (w281:bool)
              }
            }
          }
        }
      }
    }
  }
  n175 = while {
    tunnel: w31 -> [w285]
    tunnel: w30 -> [w284]
    tunnel: [w282] -> w28
    stop <- w282 stop-if-true
    # "Инициализация источников"
    n176 = Wait (ms)(milliseconds to wait=u32 1) -> ()  [unwired: 1 out]
    n177 = flat-sequence {
      tunnel: w285 -> [w328]
      tunnel: w284 -> [w327]
      tunnel: [w291] -> w282
      frame #0 {
        w303 = T4 0 items=["Current", "Voltage"] ("measurement type")
        n178 = call <instrlib>:"niDCPower Configure Current Limit.vi"("current limit"="VDD33A_curlim, A", "channel name"="0", "instrument handle"=w328) -> ("instrument handle out"=w312:refnum<k15>)  [unwired: 7 in, 1 out]
        n179 = call <instrlib>:"niDCPower Configure Current Limit.vi"("current limit"="VDD18A_curlim, A", "channel name"="1", "instrument handle"=w328) -> ("instrument handle out"=w306:refnum<k15>)  [unwired: 7 in, 1 out]
        n180 = call <instrlib>:"niDCPower Configure Current Limit.vi"("current limit"="VDD18D_curlim, A", "channel name"="0", "instrument handle"=w327) -> ("error out"=w290:errorcluster, "instrument handle out"=w307:refnum<k15>)  [unwired: 7 in]
        n181 = call <instrlib>:"niDCPower Configure Voltage Level.vi"("voltage level"="VDD33A, V", "channel name"="0", "instrument handle"=w312) -> ("error out"=w317:errorcluster, "instrument handle out"=w318:refnum<k15>)  [unwired: 7 in]
        n182 = call <instrlib>:"niDCPower Configure Voltage Level.vi"("voltage level"="VDD18A, V", "channel name"="1", "instrument handle"=w306) -> ("error out"=w315:errorcluster, "instrument handle out"=w316:refnum<k15>)  [unwired: 7 in]
        n183 = call <instrlib>:"niDCPower Configure Voltage Level.vi"("error in (no error)"=w290, "voltage level"="VDD18D, V", "channel name"="0", "instrument handle"=w307) -> ("error out"=w319:errorcluster, "instrument handle out"=w320:refnum<k15>)  [unwired: 6 in]
        n184 = call <instrlib>:"niDCPower Configure Output Enabled.vi"("error in (no error)"=w317, "output enabled"="VDD33_ON", "channel name"="0", "instrument handle"=w318) -> ("error out"=w322:errorcluster, "instrument handle out"=w321:refnum<k15>)  [unwired: 6 in]
        n185 = call <instrlib>:"niDCPower Configure Output Enabled.vi"("error in (no error)"=w315, "output enabled"="VDD18_ON", "channel name"="1", "instrument handle"=w316) -> ("error out"=w324:errorcluster, "instrument handle out"=w323:refnum<k15>)  [unwired: 6 in]
        n186 = call <instrlib>:"niDCPower Configure Output Enabled.vi"("error in (no error)"=w319, "output enabled"="VDD18_ON", "channel name"="0", "instrument handle"=w320) -> ("error out"=w326:errorcluster, "instrument handle out"=w325:refnum<k15>)  [unwired: 6 in]
        n187 = call <instrlib>:"niDCPower Measure.vi"("error in (no error)"=w322, "measurement type"=w303, "channel name"="0", "instrument handle"=w321) -> ("measurement"=→"VDD33A_cur, A" →"VDD18A_char":dbl)  [unwired: 5 in, 2 out]
        n188 = call <instrlib>:"niDCPower Measure.vi"("error in (no error)"=w324, "measurement type"=w303, "channel name"="1", "instrument handle"=w323) -> ("measurement"=→"VDD18A_cur, A" →"VD18A_char":dbl)  [unwired: 5 in, 2 out]
        n189 = call <instrlib>:"niDCPower Measure.vi"("error in (no error)"=w326, "measurement type"=w303, "channel name"="0", "instrument handle"=w325) -> ("measurement"=→"VDD18D_cur, A" →"VDD18D_char":dbl)  [unwired: 5 in, 2 out]
        n190 = local read "Power OFF"() -> (w291:bool)
      }
    }
  }
  n191 = while {
    tunnel: w3 -> [w333]
    shift-right: ["Кадр готов"] -> _
    shift-left: FALSE ("SAVE") -> [w332]
    tunnel: [w330] -> w5
    stop <- w330 stop-if-true
    n192 = Wait (ms)(milliseconds to wait=u32 1) -> ()  [unwired: 1 out]
    n193 = Greater?(x="Кадр готов", y=w332) -> (0:w329:bool)
    n194 = case shown="True" w329 {
      tunnel: w333 -> [_ w337]
      frame False {
      }
      frame True {
        n195 = local read "DataToFrame"() -> (w336:u16[][])
        n196 = local read "NumberOfAdd"() -> (w341:u32)
        n197 = To Long Integer(number=w341) -> (32bit integer=w342:i32)
        n198 = Reshape Array(w336, w342) -> (w340:u16[])
        n199 = for {
          N: 1024 -> [_]
          tunnel: w340 -> [w348]
          shift-right: [w344] -> _
          shift-left: 0 -> [w346]
          tunnel: [w347] -> w343 mode=indexing
          w345 = 1280 ("length")
          n200 = Array Subset(array=w348, index=w346, length=w345) -> (w347:u16[])
          n201 = Add(x=w345, y=w346) -> (x+y=w344:i32)
        }
        n202 = call "IMAQ ArrayToImage"("Image Pixels (U16)"=w343, "Image"=w337) -> ("Image Out"=→"Image":T1)  [unwired: 8 in, 1 out]
      }
    }
    n203 = local read "STOP"() -> (w330:bool)
  }
  n204 = while {
    tunnel: w2 -> [w366]
    tunnel: w12 -> [_]
    tunnel: w13 -> [_]
    tunnel: w15 -> [_]
    tunnel: [w365] -> w35
    tunnel: [w360] -> w27
    tunnel: w14 -> [_]
    stop <- w365 stop-if-true
    # "Инициализация переменных Target"
    n205 = Wait (ms)(milliseconds to wait=u32 1) -> ()  [unwired: 1 out]
    n206 = local read "STOP"() -> (w365:bool)
    n207 = xnode "Read/Write Control"("FPGA VI Reference In"=w366, "RESET"="RESET", "Автомат"="Автомат", "Делитель 24/x"="Делитель 24/x", "Stop_FPGA"=w365, "18_STOP"="19_STOP", "26_STOP"="27_STOP", "Такт чтения после адреса"="Такт чтения после адреса", "Чтение по С(F)/Ф(T)"="Чтение по С(F)/Ф(T)", "CSN в конце по С(F)/Ф(T)"="CSN в конце по С(F)/Ф(T)", "NumberOfAdd"="NumberOfAdd", "Request"="Request", "Retrieve"="Retrieve", "TrigTime"="TrigTime") -> ("FPGA VI Reference Out"=w360:refnum<k20>, "AddCounter"=→"AddCounter":u32, "CountFIFO"=→"CountFIFO":u32)  [unwired: 1 in, 1 out]
  }
  n208 = while {
    shift-right: ["Сохранить"] -> _
    shift-left: FALSE ("SAVE") -> [w370]
    tunnel: w3 -> [_]
    tunnel: [w367] -> w4
    stop <- w367 stop-if-true
    n209 = Wait (ms)(milliseconds to wait=u32 1) -> ()  [unwired: 1 out]
    n210 = Greater?(x="Сохранить", y=w370) -> (0:w371:bool)
    n211 = case shown="True" w371 {
      frame False {
      }
      frame True {
        n212 = local read "Образец №"() -> (w388:string)
        n213 = Concatenate Strings("Образец_" ("string"), w388) -> (w389:string)
        n214 = Build Path(base path="Frames", name or relative path=w389) -> (appended path=w396:path)
        n215 = call <vilib>:"Check if File or Folder Exists.vi"("path"=w396) -> ("file or folder exists?"=w395:bool, "dup path"=w394:path)  [unwired: 8 in, 1 out]
        n216 = case shown="False" w395 {
          tunnel: w394 -> [w401 w402]
          tunnel: [w400 w402] -> w380
          frame False {
            n217 = Create Folder(path (use dialog)=w401) -> (created path=w400:path)  [unwired: 2 in, 2 out]
          }
          frame True {
          }
        }
        n218 = Select(t="Светло", s="Темный(F)\nСветлый(T)", f="Темно") -> (s? t:f=w376:string)
        n219 = Build Path(base path=w380, name or relative path=w376) -> (appended path=w381:path)
        n220 = Get Date/Time In Seconds() -> (seconds since 1Jan1904=w393:timestamp)
        n221 = call <vilib>:"Check if File or Folder Exists.vi"("path"=w381) -> ("file or folder exists?"=w382:bool, "dup path"=w383:path)  [unwired: 8 in, 1 out]
        n222 = Format Date/Time String(time format string (%c)="%d %H.%M.%S", seconds (now)=w393) -> (date/time string=w392:string)  [unwired: 1 in]
        n223 = case shown="False" w382 {
          tunnel: w383 -> [w398 w399]
          tunnel: [w397 w399] -> w375
          frame False {
            n224 = Create Folder(path (use dialog)=w398) -> (created path=w397:path)  [unwired: 2 in, 2 out]
          }
          frame True {
          }
        }
        n225 = Concatenate Strings(w392, "_" ("string"), "Примечание", ".tiff" ("string")) -> (w374:string)
        n226 = local read "Image"() -> (w372:T1)
        n227 = Build Path(base path=w375, name or relative path=w374) -> (appended path=w373:path)
        n228 = call-poly "IMAQ Write File 2"("File Path"=w373, "Image"=w372) -> ()  [unwired: 8 in, 2 out]
      }
    }
    n229 = local read "STOP"() -> (w367:bool)
  }
  n230 = while {
    tunnel: w15 -> [_]
    tunnel: w14 -> [_]
    tunnel: w2 -> [w406]
    tunnel: [w409] -> _
    tunnel: w13 -> [w409]
    tunnel: w12 -> [_]
    shift-right: [w407] -> _
    shift-left: FALSE ("Питание") -> [w408]
    tunnel: [w404] -> w6
    tunnel: w3 -> [w403]
    stop <- w404 stop-if-true
    n231 = Wait (ms)(milliseconds to wait=u32 1) -> ()  [unwired: 1 out]
    n232 = stacked-sequence {
      tunnel: [_ w562] -> w404
      tunnel: w408 -> [w420 _]
      tunnel: ["Получить кадр" _] -> w407
      tunnel: w406 -> [w416 _]
      tunnel: w403 -> [w414 _]
      frame #0 {
        n233 = local read "FirmwareIsDone"() -> (w410:bool)
        n234 = local read "SEL"() -> (w415:bool)
        n235 = Greater?(x="Получить кадр", y=w420) -> (0:w419:bool)
        n236 = Not(x=w415) -> (.not. x?=w412:bool)
        n237 = Or(x=w419, y="Непрерывно") -> (x .or. y?=w413:bool)
        n238 = Compound Arithmetic op=AND(w410, w413, w412) -> (w411:bool)
        n239 = case shown="True" w411 {
          tunnel: w416 -> [_ w422]
          tunnel: w414 -> [_ w421]
          frame False {
          }
          frame True {
            n240 = stacked-sequence {
              tunnel: w422 -> [_ w430 w455 w488 w539]
              tunnel: w421 -> [_ _ _ _ _]
              frame #0 {
                n241 = flat-sequence {
                  frame #0 {
                    n242 = while {
                      stop <- w424 stop-if-true
                      n243 = local read "FirmwareIsDone"() -> (w424:bool)
                      n244 = Wait (ms)(milliseconds to wait=u32 1) -> ()  [unwired: 1 out]
                    }
                  }
                  frame #1 {
                    n245 = local write "DataFailure"(FALSE ("DataFailure")) -> ()
                    n246 = local write "Кадр готов"(FALSE ("Кадр готов")) -> ()
                  }
                  frame #2 {
                    n247 = Wait (ms)(milliseconds to wait=u32 1) -> ()  [unwired: 1 out]
                  }
                }
              }
              frame #1 {
                n248 = flat-sequence {
                  tunnel: w430 -> [w433]
                  tunnel: [w434] -> w429
                  tunnel: w429 -> [w437]
                  tunnel: [w435] -> w428
                  tunnel: [w440] -> w431
                  tunnel: w428 -> [w441]
                  tunnel: w431 -> [w443]
                  frame #0 {
                    n249 = xnode "Read/Write Control"("FPGA VI Reference In"=w433, "ForcedStopMemory"=TRUE) -> ("FPGA VI Reference Out"=w434:refnum<k20>)  [unwired: 1 in, 1 out]
                  }
                  frame #1 {
                    n250 = xnode "Read/Write Control"("FPGA VI Reference In"=w437, "ForcedStopMemory"=FALSE) -> ("FPGA VI Reference Out"=w436:refnum<k20>)  [unwired: 1 in, 1 out]
                    n251 = xnode "Read/Write Control"("FPGA VI Reference In"=w436, "DataToMemory"=FALSE) -> ("FPGA VI Reference Out"=w435:refnum<k20>)  [unwired: 1 in, 1 out]
                  }
                  frame #2 {
                    n252 = xnode "Read/Write Control"("FPGA VI Reference In"=w441, "ResetMemory"=TRUE ("MemoryIsDone")) -> ("FPGA VI Reference Out"=w440:refnum<k20>)  [unwired: 1 in, 1 out]
                  }
                  frame #3 {
                    n253 = xnode "Read/Write Control"("FPGA VI Reference In"=w443, "ResetMemory"=FALSE ("DataToMemory")) -> ()  [unwired: 1 in, 2 out]
                  }
                }
              }
              frame #2 {
                n254 = flat-sequence {
                  tunnel: [w458] -> w456
                  tunnel: w447 -> [w457]
                  tunnel: w456 -> [w465]
                  tunnel: [w463] -> w448
                  tunnel: [w460] -> w445
                  tunnel: w448 -> [w470]
                  tunnel: [w469] -> w446
                  tunnel: w445 -> [w468]
                  tunnel: w446 -> [w485]
                  frame #0 {
                    n255 = xnode "Read/Write Control"("FPGA VI Reference In"=w457, "DataToMemory"=TRUE) -> ("FPGA VI Reference Out"=w458:refnum<k20>)  [unwired: 1 in, 1 out]
                  }
                  frame #1 {
                    n256 = xnode "Read/Write Control"("FPGA VI Reference In"=w465, "TRIG"=TRUE) -> ("FPGA VI Reference Out"=w464:refnum<k20>)  [unwired: 1 in, 1 out]
                    n257 = xnode "Read/Write Control"("FPGA VI Reference In"=w464, "TRIG"=FALSE) -> ("FPGA VI Reference Out"=w463:refnum<k20>)  [unwired: 1 in, 1 out]
                    n258 = local read "SEL"() -> (w460:bool)
                  }
                  frame #2 {
                    n259 = local read "SEL"() -> (w466:bool)
                    n260 = Or(x=w468, y=w466) -> (x .or. y?=w467:bool)
                    n261 = while {
                      tunnel: w470 -> [w479]
                      tunnel: [w477] -> w469
                      shift-right: [w471] -> _
                      shift-left: w467 -> [w472]
                      i -> [w482]
                      stop <- w476 stop-if-true
                      n262 = xnode "Read/Write Control"("FPGA VI Reference In"=w479) -> ("MemoryIsDone"=w475:bool)  [unwired: 1 in, 2 out]
                      n263 = To Unsigned Long Integer(number=w482) -> (unsigned 32bit integer=w481:u32)
                      "DataTime" <- w481
                      n264 = case shown="True" w472 {
                        frame False {
                        }
                        frame True {
                          "DataFailure" <- TRUE ("DataFailure")
                        }
                      }
                      n265 = Greater?(x=w481, y="WatchDogTime") -> (0:w478:bool)
                      n266 = xnode "Read/Write Control"("FPGA VI Reference In"=w479, "ForcedStopMemory"=w478) -> ("FPGA VI Reference Out"=w477:refnum<k20>)  [unwired: 1 in, 1 out]
                      n267 = local read "STOP"() -> (w473:bool)
                      n268 = Or(x=w473, y=w475) -> (x .or. y?=w476:bool)
                      n269 = local read "SEL"() -> (w471:bool)
                      n270 = Wait (ms)(milliseconds to wait=u32 1) -> ()  [unwired: 1 out]
                    }
                  }
                  frame #3 {
                    n271 = xnode "Read/Write Control"("FPGA VI Reference In"=w485, "ForcedStopMemory"=FALSE) -> ()  [unwired: 1 in, 2 out]
                  }
                }
                n272 = xnode "Invoke Method"("FPGA VI Reference In"=w455, "Number of Elements"=u32 0, "Timeout (ms)"=0) -> ("FPGA VI Reference Out"=w454:refnum<k20>, "error out"=w449:errorcluster, "Elements Remaining"=w451:u32)  [unwired: 1 in, 1 out]
                n273 = xnode "Invoke Method"("FPGA VI Reference In"=w454, "error in"=w449, "Number of Elements"=w451, "Timeout (ms)"=0) -> ("FPGA VI Reference Out"=w447:refnum<k20>)  [unwired: 3 out]
              }
              frame #3 {
                n274 = for {
                  N: 16 -> [_]
                  shift-right: [w494] -> _
                  shift-left: u32 0 -> [w495]
                  shift-right: [w493] -> _
                  shift-left: u32 81920 -> [w492]
                  tunnel: w488 -> [w497]
                  tunnel: [w496] -> w486 mode=indexing
                  i -> [w491]
                  n275 = stacked-sequence {
                    tunnel: w497 -> [w503 w504 w516 w532]
                    tunnel: [_ _ _ w531] -> w496
                    tunnel: w495 -> [w501 _ _ _]
                    tunnel: w492 -> [w498 _ _ _]
                    tunnel: [w500 _ _ _] -> w494
                    tunnel: [w502 _ _ _] -> w493
                    tunnel: w491 -> [_ _ _ _]
                    frame #0 {
                      w499 = u32 81920
                      n276 = xnode "Read/Write Control"("FPGA VI Reference In"=w503, "FirstAdd"=w501, "LastAdd"=w498) -> ()  [unwired: 1 in, 2 out]
                      n277 = Add(x=w501, y=w499) -> (x+y=w500:u32)
                      n278 = Add(x=w499, y=w498) -> (x+y=w502:u32)
                    }
                    frame #1 {
                      n279 = flat-sequence {
                        tunnel: w504 -> [w508]
                        tunnel: [w507] -> w506
                        tunnel: w506 -> [w511]
                        tunnel: [w510] -> w505
                        tunnel: w505 -> [w513]
                        frame #0 {
                          n280 = xnode "Read/Write Control"("FPGA VI Reference In"=w508, "MemoryToFIFO"=FALSE) -> ("FPGA VI Reference Out"=w507:refnum<k20>)  [unwired: 1 in, 1 out]
                        }
                        frame #1 {
                          n281 = xnode "Read/Write Control"("FPGA VI Reference In"=w511, "ResetFIFO"=TRUE) -> ("FPGA VI Reference Out"=w510:refnum<k20>)  [unwired: 1 in, 1 out]
                        }
                        frame #2 {
                          n282 = xnode "Read/Write Control"("FPGA VI Reference In"=w513, "ResetFIFO"=FALSE) -> ()  [unwired: 1 in, 2 out]
                        }
                      }
                    }
                    frame #2 {
                      n283 = xnode "Read/Write Control"("FPGA VI Reference In"=w516, "MemoryToFIFO"=TRUE) -> ("FPGA VI Reference Out"=w515:refnum<k20>)  [unwired: 1 in, 1 out]
                      n284 = while {
                        tunnel: w515 -> [w530]
                        tunnel: [w529] -> _
                        i -> [w528]
                        stop <- w524 stop-if-true
                        n285 = local read "WatchDogTime"() -> (w519:u32)
                        n286 = local read "DataTime"() -> (w520:u32)
                        n287 = xnode "Read/Write Control"("FPGA VI Reference In"=w530) -> ("FPGA VI Reference Out"=w529:refnum<k20>, "FIFOIsDone"=w522:bool)  [unwired: 1 in, 1 out]
                        n288 = To Unsigned Long Integer(number=w528) -> (unsigned 32bit integer=w527:u32)
                        n289 = Greater?(x=w527, y=u32 1000) -> (0:w521:bool)
                        n290 = Greater Or Equal?(x=w520, y=w519) -> ()  [unwired: 1 out]
                        n291 = Wait (ms)(milliseconds to wait=u32 1) -> ()  [unwired: 1 out]
                        n292 = Compound Arithmetic op=OR(w522, w521) -> (w518:bool)
                        n293 = local read "STOP"() -> (w523:bool)
                        n294 = Or(x=w518, y=w523) -> (x .or. y?=w524:bool)
                      }
                    }
                    frame #3 {
                      n295 = xnode "Invoke Method"("FPGA VI Reference In"=w532, "Number of Elements"=u32 0, "Timeout (ms)"=0) -> ("FPGA VI Reference Out"=w538:refnum<k20>, "error out"=w536:errorcluster, "Elements Remaining"=w537:u32)  [unwired: 1 in, 1 out]
                      n296 = xnode "Invoke Method"("FPGA VI Reference In"=w538, "error in"=w536, "Number of Elements"=w537, "Timeout (ms)"=0) -> ("Data"=w531:u16[])  [unwired: 3 out]
                    }
                  }
                }
                "DataToFrame" <- w486
              }
              frame #4 {
                n297 = flat-sequence {
                  tunnel: w539 -> [w548]
                  frame #0 {
                    n298 = xnode "Read/Write Control"("FPGA VI Reference In"=w548) -> ("NumberOfAdd"=w547:u32)  [unwired: 1 in, 2 out]
                    n299 = local read "AddCounter"() -> (w546:u32)
                    n300 = Not Equal?(x=w547, y=w546) -> (x != y?=w545:bool)
                    n301 = Select(t=TRUE ("Кадр готов"), s=w545, f=FALSE ("Кадр готов")) -> (s? t:f=w542:bool)
                    n302 = Not(x=w542) -> (.not. x?=w541:bool)
                    n303 = local write "Кадр готов"(w541) -> ()
                    n304 = Wait (ms)(milliseconds to wait=u32 1) -> ()  [unwired: 1 out]
                  }
                  frame #1 {
                    # "Время выполнения кода после получения кадра почти 500 мс. Этого хватает до значения в 14м регистре 7900, дальше нужна задержка 1,5*DataTime времени получения данных в DataToFrame  +  запас по времени,т.е. 3,2*(DataTime/3)"
                    # "Параметрическая задержка"
                    n305 = local read "DataTime"() -> (w561:u32)
                    n306 = Divide(x=w561, y=u32 2) -> (x/y=w558:dbl)
                    n307 = Multiply(x=w558, y=3.2) -> (x*y=w559:dbl)
                    n308 = To Unsigned Long Integer(number=w559) -> (unsigned 32bit integer=w554:u32)
                    n309 = local read "DataFailure"() -> (w551:bool)
                    n310 = Greater?(x=w554, y=u32 500) -> (0:w555:bool)
                    n311 = Select(t=w554, s=w555, f=u32 0) -> (s? t:f=w552:u32)
                    n312 = Select(t=u32 0, s=w551, f=w552) -> (s? t:f=w549:u32)
                    "DelayFrame" <- w549
                    n313 = Wait (ms)(milliseconds to wait=w549) -> ()  [unwired: 1 out]
                  }
                }
              }
            }
          }
        }
      }
      frame #1 {
        n314 = local read "STOP"() -> (w562:bool)
      }
    }
  }
  n315 = while {
    tunnel: [w576] -> w20
    tunnel: w2 -> [w574]
    tunnel: w15 -> [_]
    tunnel: w13 -> [_]
    tunnel: w12 -> [_]
    shift-right: [w577] -> _
    shift-left: u8 0 ("milliseconds to wait") -> [w567]
    tunnel: w14 -> [w579]
    tunnel: [w578] -> w16
    shift-right: [w563] -> _
    shift-left: FALSE ("Питание") -> [w565]
    stop <- w576 stop-if-true
    n316 = Wait (ms)(milliseconds to wait=u32 1) -> ()  [unwired: 1 out]
    n317 = local read "SEL"() -> (w563:bool)
    n318 = local read "RESET"() -> (w583:bool)
    n319 = local read "VDD33_ON"() -> (w582:bool)
    n320 = local read "FirmwareIsDone"() -> (w581:bool)
    n321 = Not(x=w563) -> (.not. x?=w573:bool)
    n322 = Search 1D Array(1D array="Маска номера", element=w567, start index (0)=0) -> (index of element=w572:i32)
    n323 = Greater?(x=w563, y=w565) -> (0:w564:bool)
    n324 = Greater?(x=w572, y=-1) -> (0:w568:bool)
    n325 = Compound Arithmetic op=AND("Проверка\nсбоев", w573, w583, w582, w581) -> (w580:bool)
    n326 = case shown="True" w580 {
      tunnel: [u8 0 ("milliseconds to wait") w604] -> w577
      tunnel: w579 -> [w591 w613]
      tunnel: [w591 w612] -> w578
      tunnel: [w589 w607] -> w576
      tunnel: w567 -> [_ w606]
      tunnel: w574 -> [w585 w605]
      tunnel: w568 -> [_ w603]
      tunnel: w564 -> [w588 _]
      tunnel: "Проверка\nсбоев" -> [w587 _]
      frame False {
        n327 = And(x=w588, y=w587) -> (x .and. y?=w586:bool)
        n328 = case shown="True" w586 {
          tunnel: w585 -> [_ w592]
          frame False {
          }
          frame True {
            n329 = flat-sequence {
              tunnel: w592 -> [w599]
              frame #0 {
                n330 = while {
                  stop <- w594 stop-if-true
                  n331 = local read "FirmwareIsDone"() -> (w597:bool)
                  n332 = local read "SEL"() -> (w596:bool)
                  n333 = Not(x=w596) -> (.not. x?=w595:bool)
                  n334 = Wait (ms)(milliseconds to wait=u32 1) -> ()  [unwired: 1 out]
                  n335 = And(x=w595, y=w597) -> (x .and. y?=w594:bool)
                }
              }
              frame #1 {
                n336 = xnode "Read/Write Control"("FPGA VI Reference In"=w599, "TRIG"=TRUE) -> ("FPGA VI Reference Out"=w602:refnum<k20>)  [unwired: 1 in, 1 out]
                n337 = Wait (ms)(milliseconds to wait=u32 5) -> ()  [unwired: 1 out]
                n338 = xnode "Read/Write Control"("FPGA VI Reference In"=w602, "TRIG"=FALSE) -> ()  [unwired: 1 in, 2 out]
              }
            }
          }
        }
        n339 = local write "Сбой"(FALSE ("Был сбой")) -> ()
        n340 = local read "STOP"() -> (w589:bool)
      }
      frame True {
        n341 = Equal?(x=w606, y=u8 127) -> (x = y?=w608:bool)
        n342 = case shown="True" w603 {
          tunnel: w613 -> [w614 w621]
          tunnel: [w614 w620] -> w612
          tunnel: w608 -> [_ w619]
          tunnel: [w615 w618] -> w607
          tunnel: w606 -> [_ w617]
          tunnel: w605 -> [_ w616]
          frame False {
            n343 = local read "STOP"() -> (w615:bool)
          }
          frame True {
            n344 = stacked-sequence {
              seq-local: [w624 _ _] -> [_ w645 _]
              tunnel: w621 -> [_ w648 _]
              tunnel: [_ w647 _] -> w620
              tunnel: w619 -> [_ _ w677]
              tunnel: [_ _ w676] -> w618
              tunnel: w617 -> [w622 w644 _]
              tunnel: w616 -> [w623 _ w674]
              frame #0 {
                n345 = flat-sequence {
                  tunnel: w622 -> [w630]
                  tunnel: [w638] -> w624
                  tunnel: w623 -> [w639]
                  frame #0 {
                    n346 = while {
                      stop <- w628 stop-if-true
                      n347 = local read "SPI_Read"() -> (w629:bool)
                      n348 = local read "STOP"() -> (w626:bool)
                      n349 = Not(x=w629) -> (.not. x?=w627:bool)
                      n350 = Or(x=w626, y=w627) -> (x .or. y?=w628:bool)
                      n351 = Wait (ms)(milliseconds to wait=u32 1) -> ()  [unwired: 1 out]
                    }
                  }
                  frame #1 {
                    n352 = To Unsigned Byte Integer(number=w630) -> (unsigned 8bit integer=w632:u8)
                    n353 = local write "ReadIsDone"(FALSE ("ReadIsDone")) -> ()
                    n354 = local write "RegForRead"(w632) -> ()
                  }
                  frame #2 {
                    n355 = local write "SPI_Read"(TRUE ("SPI_Read")) -> ()
                  }
                  frame #3 {
                    n356 = while {
                      stop <- w636 stop-if-true
                      n357 = local read "ReadIsDone"() -> (w634:bool)
                      n358 = local read "STOP"() -> (w635:bool)
                      n359 = Or(x=w635, y=w634) -> (x .or. y?=w636:bool)
                      n360 = Wait (ms)(milliseconds to wait=u32 1) -> ()  [unwired: 1 out]
                    }
                  }
                  frame #4 {
                    n361 = xnode "Read/Write Control"("FPGA VI Reference In"=w639) -> ("MISO"=w640:bool[])  [unwired: 1 in, 2 out]
                    n362 = Boolean Array To Number(Boolean array=w640) -> (number=w638:u16)
                  }
                }
              }
              frame #1 {
                n363 = local read "Содержание всех регистров"() -> (w643:u16[])
                n364 = local read "FirmwareIsDone"() -> (w650:bool)
                n365 = local read "RESET"() -> (w651:bool)
                n366 = local read "SEL"() -> (w642:bool)
                n367 = Index Array(array=w643, index=w644) -> (element=w646:u16)
                n368 = Not(x=w642) -> (.not. x?=w641:bool)
                n369 = Not Equal?(x=w646, y=w645) -> (x != y?=w649:bool)
                n370 = Compound Arithmetic op=AND(w649, w651, w650, w641) -> (w652:bool)
                n371 = case shown="True" w652 {
                  tunnel: w644 -> [_ w672]
                  tunnel: w645 -> [_ w671]
                  tunnel: w646 -> [_ w667]
                  tunnel: w648 -> [w653 w661]
                  tunnel: [w653 w660] -> w647
                  frame False {
                  }
                  frame True {
                    w658 = i16 0 ("width (-)")
                    w657 = "\t"
                    # "Номер сбоя"
                    # "Данные default"
                    # "Данные при сбое"
                    # "Номер регистра"
                    # "Дата и время"
                    n372 = local read "Счетчик сбоев"() -> (w673:u16)
                    n373 = Increment(x=w673) -> (x+1=w664:u16)
                    "Счетчик сбоев" <- w664
                    n374 = Number To Fractional String(number=w672, precision (6)=w658) -> (F-format string=w670:string)  [unwired: 2 in]
                    "№" <- w670
                    n375 = Number To Fractional String(number=w671, precision (6)=w658) -> (F-format string=w669:string)  [unwired: 2 in]
                    "During SEU" <- w669
                    n376 = Number To Fractional String(number=w667, precision (6)=w658) -> (F-format string=w668:string)  [unwired: 2 in]
                    "Default" <- w668
                    n377 = Get Date/Time In Seconds() -> (seconds since 1Jan1904=w663:timestamp)
                    n378 = Number To Fractional String(number=w664, precision (6)=w658) -> (F-format string=w666:string)  [unwired: 2 in]
                    n379 = Format Date/Time String(time format string (%c)="%d %H:%M:%S:%3u", seconds (now)=w663) -> (date/time string=w654:string)  [unwired: 1 in]
                    "Last SEU Time" <- w654
                    n380 = Concatenate Strings(w657, w670, w657, w669, w657, w668, w657, w666, "\r\n") -> (w655:string)
                    n381 = Concatenate Strings(w654, w655) -> (w656:string)
                    n382 = Format Into String(initial string=w661, w656) -> (resulting string=w660:refnum<file>)  [unwired: 2 in, 1 out]
                    "Сбой" <- TRUE ("Был сбой")
                  }
                }
              }
              frame #2 {
                n383 = local read "Сбой"() -> (w675:bool)
                n384 = And(x=w675, y=w677) -> (x .and. y?=w678:bool)
                n385 = case shown="True" w678 {
                  tunnel: [w679 w684] -> w676
                  tunnel: w674 -> [_ w683]
                  frame False {
                    n386 = local read "STOP"() -> (w679:bool)
                  }
                  frame True {
                    n387 = flat-sequence {
                      tunnel: w683 -> [w685]
                      tunnel: [w685] -> w681
                      tunnel: [w688] -> w682
                      tunnel: w681 -> [w688]
                      tunnel: w682 -> [w694]
                      tunnel: [w691] -> w680
                      tunnel: [w704] -> w684
                      tunnel: w680 -> [_]
                      frame #0 {
                        n388 = local write "RESET"(FALSE ("RESET")) -> ()
                        n389 = Wait (ms)(milliseconds to wait=u32 5) -> ()  [unwired: 1 out]
                      }
                      frame #1 {
                        n390 = local write "RESET"(TRUE ("RESET")) -> ()
                        n391 = Wait (ms)(milliseconds to wait=u32 5) -> ()  [unwired: 1 out]
                      }
                      frame #2 {
                        n392 = while {
                          tunnel: w694 -> [w700]
                          tunnel: [w700] -> w693
                          stop <- w698 stop-if-true
                          n393 = local read "FirmwareIsDone"() -> (w699:bool)
                          n394 = local read "STOP"() -> (w697:bool)
                          n395 = Wait (ms)(milliseconds to wait=u32 1) -> ()  [unwired: 1 out]
                          n396 = Or(x=w697, y=w699) -> (x .or. y?=w698:bool)
                        }
                        n397 = xnode "Read/Write Control"("FPGA VI Reference In"=w693, "TRIG"=TRUE) -> ("FPGA VI Reference Out"=w692:refnum<k20>)  [unwired: 1 in, 1 out]
                        n398 = xnode "Read/Write Control"("FPGA VI Reference In"=w692, "TRIG"=FALSE) -> ("FPGA VI Reference Out"=w691:refnum<k20>)  [unwired: 1 in, 1 out]
                      }
                      frame #3 {
                        n399 = local read "STOP"() -> (w704:bool)
                        n400 = Wait (ms)(milliseconds to wait=u32 1) -> ()  [unwired: 1 out]
                        n401 = local write "Сбой"(FALSE ("Был сбой")) -> ()
                      }
                    }
                  }
                }
              }
            }
          }
        }
        n402 = Increment(x=w606) -> (x+1=w609:u8)
        n403 = Select(t=u8 0 ("f"), s=w608, f=w609) -> (s? t:f=w604:u8)
      }
    }
    "Reg Counter" <- w567
  }
  n404 = while {
    shift-right: ["SPI_Read"] -> _
    shift-left: FALSE ("Питание") -> [w710]
    tunnel: w2 -> [w709]
    tunnel: w15 -> [_]
    tunnel: w13 -> [_]
    tunnel: w12 -> [_]
    tunnel: [w706] -> w23
    tunnel: [w707] -> _
    tunnel: w14 -> [w707]
    stop <- w706 stop-if-true
    # "SPI чтение"
    n405 = Wait (ms)(milliseconds to wait=u32 1) -> ()  [unwired: 1 out]
    n406 = Greater?(x="SPI_Read", y=w710) -> (0:w711:bool)
    n407 = case shown="True" w711 {
      tunnel: w709 -> [_ w719]
      tunnel: [w712 w713] -> w706
      frame False {
        n408 = local read "STOP"() -> (w712:bool)
      }
      frame True {
        n409 = flat-sequence {
          tunnel: w719 -> [w728]
          tunnel: [w729] -> w717
          tunnel: [w726] -> w715
          tunnel: w717 -> [w742]
          tunnel: [w741] -> w716
          tunnel: w715 -> [w743]
          tunnel: w716 -> [w746]
          tunnel: [w744] -> w714
          tunnel: [w760] -> w718
          tunnel: w714 -> [w756]
          tunnel: w718 -> [w763]
          frame #0 {
            # "Последний бит - чтение"
            n410 = Number To Boolean Array(number="RegForRead") -> (Boolean array=w740:bool[])
            n411 = local write "SPI_Read"(FALSE ("SPI_Read")) -> ()
            n412 = Greater?(x="RegForRead", y=u8 3) -> (0:w727:bool)
            n413 = Number To Boolean Array(number=u16 0 ("index")) -> (Boolean array=w733:bool[])
            n414 = Delete From Array(array=w733, length=8) -> (array with subset deleted=w731:bool[])  [unwired: 1 in, 1 out]
            n415 = Replace Array Subset(array=w740, new element=FALSE ("new element/subarray"), index=7) -> (w725:bool[])
            n416 = Select(t=w733, s=w727, f=w731) -> (s? t:f=w724:bool[])
            n417 = xnode "Read/Write Control"("FPGA VI Reference In"=w728, "8-bit(F)/16-bit(T)"=w727) -> ("FPGA VI Reference Out"=w726:refnum<k20>)  [unwired: 1 in, 1 out]
            n418 = local write "ReadIsDone"(FALSE ("ReadIsDone")) -> ()
            n419 = Insert Into Array(array=w724, index=16, new element=w725) -> (w730:bool[])
            n420 = Insert Into Array(array=w724, index=8, new element=w725) -> (w723:bool[])
            n421 = Select(t=w730, s=w727, f=w723) -> (s? t:f=w729:bool[])
          }
          frame #1 {
            n422 = xnode "Read/Write Control"("FPGA VI Reference In"=w743, "MOSI"=w742) -> ("FPGA VI Reference Out"=w741:refnum<k20>)  [unwired: 1 in, 1 out]
            n423 = local write "MOSI"(w742) -> ()
          }
          frame #2 {
            w747 = TRUE ("SPI")
            n424 = xnode "Read/Write Control"("FPGA VI Reference In"=w746, "SPI"=w747) -> ("FPGA VI Reference Out"=w745:refnum<k20>)  [unwired: 1 in, 1 out]
            n425 = while {
              tunnel: w745 -> [w753]
              tunnel: [w751] -> w744
              stop <- w750 stop-if-true
              n426 = local read "STOP"() -> (w748:bool)
              n427 = xnode "Read/Write Control"("FPGA VI Reference In"=w753) -> ("FPGA VI Reference Out"=w751:refnum<k20>, "SPI_is_done"=w749:bool)  [unwired: 1 in, 1 out]
              n428 = Or(x=w749, y=w748) -> (x .or. y?=w750:bool)
              n429 = Wait (ms)(milliseconds to wait=u32 1) -> ()  [unwired: 1 out]
            }
            n430 = local write "SPI"(w747) -> ()
          }
          frame #3 {
            w758 = FALSE ("SPI")
            n431 = xnode "Read/Write Control"("FPGA VI Reference In"=w756) -> ("FPGA VI Reference Out"=w757:refnum<k20>, "MISO"=w755:bool[])  [unwired: 1 in, 1 out]
            n432 = xnode "Read/Write Control"("FPGA VI Reference In"=w757, "SPI"=w758) -> ("FPGA VI Reference Out"=w759:refnum<k20>)  [unwired: 1 in, 1 out]
            n433 = xnode "Read/Write Control"("FPGA VI Reference In"=w759, "ResetSPI"=TRUE ("SPI_is_done")) -> ("FPGA VI Reference Out"=w760:refnum<k20>)  [unwired: 1 in, 1 out]
            n434 = local write "SPI"(w758) -> ()
            n435 = Boolean Array To Number(Boolean array=w755) -> (number=→"DataRead":u16)
            n436 = local write "MISO"(w755) -> ()
          }
          frame #4 {
            n437 = xnode "Read/Write Control"("FPGA VI Reference In"=w763, "ResetSPI"=FALSE ("SPI_is_done")) -> ()  [unwired: 1 in, 2 out]
            "ReadIsDone" <- TRUE ("ReadIsDone")
          }
        }
        n438 = local read "STOP"() -> (w713:bool)
      }
    }
  }
  n439 = while {
    tunnel: w12 -> [_]
    tunnel: w13 -> [_]
    tunnel: w2 -> [w767]
    tunnel: w15 -> [_]
    tunnel: [w766] -> w34
    shift-right: ["SPI_Write"] -> _
    shift-left: FALSE ("Питание") -> [w770]
    tunnel: w14 -> [_]
    stop <- w766 stop-if-true
    # "SPI запись"
    n440 = Wait (ms)(milliseconds to wait=u32 1) -> ()  [unwired: 1 out]
    n441 = Greater?(x="SPI_Write", y=w770) -> (0:w768:bool)
    n442 = case shown="True" w768 {
      tunnel: w767 -> [_ w778]
      tunnel: [w771 w773] -> w766
      frame False {
        n443 = local read "STOP"() -> (w771:bool)
      }
      frame True {
        n444 = flat-sequence {
          tunnel: w778 -> [w785]
          tunnel: [w784] -> w777
          tunnel: [w782] -> w775
          tunnel: w777 -> [w802]
          tunnel: [w801] -> w776
          tunnel: w775 -> [w800]
          tunnel: w776 -> [w806]
          tunnel: [w803] -> w774
          tunnel: w774 -> [w815]
          tunnel: [w813] -> w772
          tunnel: w772 -> [w820]
          frame #0 {
            # "Последний бит - запись"
            n445 = Number To Boolean Array(number="RegForWrite") -> (Boolean array=w798:bool[])
            n446 = Number To Boolean Array(number="DataWrite") -> (Boolean array=w799:bool[])
            n447 = Greater?(x="RegForWrite", y=u8 3) -> (0:w783:bool)
            n448 = local write "SPI_Write"(FALSE ("SPI_Write")) -> ()
            n449 = Delete From Array(array=w799, length=8) -> (array with subset deleted=w797:bool[])  [unwired: 1 in, 1 out]
            n450 = Replace Array Subset(array=w798, new element=TRUE ("new element/subarray"), index=7) -> (w790:bool[])
            n451 = xnode "Read/Write Control"("FPGA VI Reference In"=w785, "8-bit(F)/16-bit(T)"=w783) -> ("FPGA VI Reference Out"=w784:refnum<k20>)  [unwired: 1 in, 1 out]
            n452 = Select(t=w799, s=w783, f=w797) -> (s? t:f=w781:bool[])
            n453 = Insert Into Array(array=w781, index=16, new element=w790) -> (w789:bool[])
            n454 = local write "WriteIsDone"(FALSE ("WriteIsDone")) -> ()
            n455 = Insert Into Array(array=w781, index=8, new element=w790) -> (w788:bool[])
            n456 = Select(t=w789, s=w783, f=w788) -> (s? t:f=w782:bool[])
          }
          frame #1 {
            n457 = xnode "Read/Write Control"("FPGA VI Reference In"=w802, "MOSI"=w800) -> ("FPGA VI Reference Out"=w801:refnum<k20>)  [unwired: 1 in, 1 out]
            n458 = local write "MOSI"(w800) -> ()
          }
          frame #2 {
            w805 = TRUE ("SPI")
            n459 = xnode "Read/Write Control"("FPGA VI Reference In"=w806, "SPI"=w805) -> ("FPGA VI Reference Out"=w804:refnum<k20>)  [unwired: 1 in, 1 out]
            n460 = while {
              tunnel: w804 -> [w812]
              tunnel: [w810] -> w803
              stop <- w809 stop-if-true
              n461 = local read "STOP"() -> (w807:bool)
              n462 = xnode "Read/Write Control"("FPGA VI Reference In"=w812) -> ("FPGA VI Reference Out"=w810:refnum<k20>, "SPI_is_done"=w808:bool)  [unwired: 1 in, 1 out]
              n463 = Or(x=w808, y=w807) -> (x .or. y?=w809:bool)
              n464 = Wait (ms)(milliseconds to wait=u32 1) -> ()  [unwired: 1 out]
            }
            n465 = local write "SPI"(w805) -> ()
          }
          frame #3 {
            w816 = FALSE ("SPI")
            n466 = xnode "Read/Write Control"("FPGA VI Reference In"=w815, "SPI"=w816) -> ("FPGA VI Reference Out"=w814:refnum<k20>)  [unwired: 1 in, 1 out]
            n467 = xnode "Read/Write Control"("FPGA VI Reference In"=w814, "ResetSPI"=TRUE ("SPI_is_done")) -> ("FPGA VI Reference Out"=w813:refnum<k20>)  [unwired: 1 in, 1 out]
            n468 = local write "SPI"(w816) -> ()
          }
          frame #4 {
            n469 = xnode "Read/Write Control"("FPGA VI Reference In"=w820, "ResetSPI"=FALSE ("SPI_is_done")) -> ()  [unwired: 1 in, 2 out]
            "WriteIsDone" <- TRUE ("Reg_W_OK")
          }
        }
        n470 = local read "STOP"() -> (w773:bool)
      }
    }
  }
  n471 = while {
    shift-right: ["TRIG"] -> _
    shift-left: FALSE ("Питание") -> [w825]
    tunnel: w15 -> [_]
    tunnel: w2 -> [w823]
    tunnel: [w821] -> w22
    tunnel: w14 -> [_]
    stop <- w821 stop-if-true
    n472 = Wait (ms)(milliseconds to wait=u32 1) -> ()  [unwired: 1 out]
    n473 = Greater?(x="TRIG", y=w825) -> (0:w826:bool)
    n474 = case shown="True" w826 {
      tunnel: w823 -> [_ w830]
      tunnel: [w827 w829] -> w821
      frame False {
        n475 = local read "STOP"() -> (w827:bool)
      }
      frame True {
        n476 = flat-sequence {
          tunnel: w830 -> [w832]
          tunnel: [w831] -> w828
          tunnel: w828 -> [w835]
          tunnel: [w834] -> _
          frame #0 {
            n477 = xnode "Read/Write Control"("FPGA VI Reference In"=w832, "TRIG"=TRUE) -> ("FPGA VI Reference Out"=w831:refnum<k20>)  [unwired: 1 in, 1 out]
          }
          frame #1 {
            n478 = xnode "Read/Write Control"("FPGA VI Reference In"=w835, "TRIG"=FALSE) -> ("FPGA VI Reference Out"=w834:refnum<k20>)  [unwired: 1 in, 1 out]
          }
        }
        n479 = local read "STOP"() -> (w829:bool)
      }
    }
  }
  n480 = while {
    tunnel: w2 -> [w840]
    tunnel: w15 -> [_]
    tunnel: w13 -> [_]
    tunnel: w12 -> [_]
    shift-right: [w842] -> _
    shift-left: FALSE ("Питание") -> [w845]
    shift-right: ["Прошить\nрегистры"] -> _
    shift-left: FALSE ("Питание") -> [w844]
    tunnel: [w841] -> w21
    tunnel: w14 -> [_]
    stop <- w841 stop-if-true
    # "Прошивка используемых для записи регистров"
    n481 = local read "RESET"() -> (w842:bool)
    n482 = Wait (ms)(milliseconds to wait=u32 1) -> ()  [unwired: 1 out]
    n483 = Greater?(x="Прошить\nрегистры", y=w844) -> (0:w839:bool)
    n484 = Greater?(x=w842, y=w845) -> (0:w838:bool)
    n485 = Or(x=w839, y=w838) -> (x .or. y?=w837:bool)
    n486 = case shown="True" w837 {
      tunnel: [w847 w849] -> w841
      tunnel: w840 -> [_ w848]
      frame False {
        n487 = local read "STOP"() -> (w847:bool)
      }
      frame True {
        n488 = stacked-sequence {
          tunnel: w848 -> [_ _ _]
          frame #0 {
            n489 = flat-sequence {
              frame #0 {
                n490 = local write "Прошить\nрегистры"(FALSE ("Прошить\nрегистры")) -> ()
                "FirmwareIsDone" <- FALSE ("FirmwareIsDone")
              }
              frame #1 {
                n491 = Wait (ms)(milliseconds to wait=u32 10) -> ()  [unwired: 1 out]
              }
            }
          }
          frame #1 {
            # "Тут данные регистров"
            n492 = Array Size(array="Номера для Записи") -> (size(s)=w855:i32)
            n493 = for {
              N: w855 -> [_]
              tunnel: "Номера для Записи" -> [w857]
              tunnel: "Регистры для записи" -> [w856]
              i -> [w858]
              n494 = flat-sequence {
                tunnel: w858 -> [w868]
                tunnel: w857 -> [w867]
                tunnel: w856 -> [w866]
                frame #0 {
                  n495 = Index Array(array=w866, index=w868) -> (element=w865:u16)
                  n496 = Index Array(array=w867, index=w868) -> (element=w860:u32)
                  n497 = To Unsigned Word Integer(number=w865) -> (unsigned 16bit integer=w862:u16)
                  n498 = local write "DataWrite"(w862) -> ()
                  n499 = To Unsigned Byte Integer(number=w860) -> (unsigned 8bit integer=w864:u8)
                  n500 = local write "RegForWrite"(w864) -> ()
                  n501 = To Long Integer(number=w860) -> (32bit integer=w861:i32)
                  n502 = Replace Array Subset(array="Содержание всех регистров", new element=w862, index=w861) -> (w863:u16[])
                  n503 = local write "Содержание всех регистров"(w863) -> ()
                }
                frame #1 {
                  n504 = local write "WriteIsDone"(FALSE ("WriteIsDone")) -> ()
                }
                frame #2 {
                  n505 = local write "SPI_Write"(TRUE ("SPI_Write")) -> ()
                }
                frame #3 {
                  n506 = while {
                    stop <- w873 stop-if-true
                    n507 = local read "STOP"() -> (w871:bool)
                    n508 = local read "WriteIsDone"() -> (w872:bool)
                    n509 = Or(x=w872, y=w871) -> (x .or. y?=w873:bool)
                    n510 = Wait (ms)(milliseconds to wait=u32 1) -> ()  [unwired: 1 out]
                  }
                }
              }
            }
          }
          frame #2 {
            n511 = local write "FirmwareIsDone"(TRUE ("FirmwareIsDone")) -> ()
          }
        }
        n512 = local read "STOP"() -> (w849:bool)
      }
    }
  }
  n513 = flat-sequence {
    tunnel: w44 -> [_]
    tunnel: w43 -> [w881]
    tunnel: w8 -> [w880]
    tunnel: w7 -> [w879]
    tunnel: w29 -> [_]
    tunnel: w35 -> [_]
    tunnel: w34 -> [_]
    tunnel: w23 -> [_]
    tunnel: w28 -> [_]
    tunnel: w27 -> [w878]
    tunnel: w22 -> [_]
    tunnel: w21 -> [_]
    tunnel: w20 -> [_]
    tunnel: w16 -> [w877]
    tunnel: w6 -> [_]
    tunnel: [w876] -> _
    tunnel: w5 -> [w876]
    tunnel: w4 -> [_]
    frame #0 {
      # "STOP"
      n514 = call <instrlib>:"niDCPower Close.vi"("instrument handle"=w880) -> ()  [unwired: 10 in, 1 out]
      n515 = call <instrlib>:"niDCPower Close.vi"("instrument handle"=w879) -> ()  [unwired: 10 in, 1 out]
      n516 = xnode "Close FPGA VI Reference"("FPGA VI Reference In"=w878) -> ()  [unwired: 1 in, 1 out]
      n517 = Close File(refnum=w881) -> ()  [unwired: 1 in, 2 out]
      n518 = Close File(refnum=w877) -> ()  [unwired: 1 in, 2 out]
    }
  }
  n519 = disable-structure shown="Disabled" {
    frame Disabled {
      n520 = xnode "Read/Write Control"("ForcedStopMemory"=TRUE) -> ("FPGA VI Reference Out"=w886:refnum<k20>, "error out"=w887:errorcluster)  [unwired: 2 in]
      n521 = xnode "Read/Write Control"("FPGA VI Reference In"=w886, "error in"=w887, "ForcedStopMemory"=FALSE) -> ("FPGA VI Reference Out"=w888:refnum<k20>, "error out"=w889:errorcluster)
      n522 = xnode "Read/Write Control"("FPGA VI Reference In"=w888, "error in"=w889, "DataToMemory"=FALSE) -> ("FPGA VI Reference Out"=w890:refnum<k20>, "error out"=w891:errorcluster)
      n523 = xnode "Read/Write Control"("FPGA VI Reference In"=w890, "error in"=w891, "MemoryToFIFO"=FALSE) -> ()  [unwired: 2 out]
    }
    frame Enabled {
    }
  }
